vi "Edit_BSA_IP.vi"(3 "Show Panel":bool) -> (1 "Run LDA Diagnostic Out":bool)   [LabVIEW 2017]
uses:
  Controls/Beam_Power.ctl
  BSA_Type.ctl
  File/Setup_Filetype.ctl
  Globals/LDA_meas_global_2.vi
  Globals/LDA_meas_global_1.vi
  Globals/Constants_global.vi
  Globals/Meas_global.vi
panel:
  out "Setup String to read":string
  out "Blue Wavelength":dbl format="%.2f"
  out "Green Wavelength":dbl format="%.2f"
  in  "BSA Type":T1
  in  "45 Degree Mirror":bool
  in  "Beam Alignment":u16(ring) items=["No Info", "Tunnel", "Model"]
  in  "Warn if Power below (mW)":T2
  out "Probe Options":string[](array[string])
  out "Green Fibre Separation":dbl[](array[numeric])
  out "Blue Fibre Separation":dbl[](array[numeric])
  in  "Cluster":cluster{"Focal Lengths":string[]}
  out "Focal Lengths Cluster":cluster{"Focal Lengths":string[]}[](array[cluster])
  out "Channel Values":string[][](array[string])
  out "Channel Names":string[](array[string])
  out "LDA_Probe_Information File":path
  in  "Focal Length 1":u16(ring) items=["160", "300"]
  in  "Focal Length 0":u16(ring) items=["160", "300"]
  in  "Non-coincident":bool=TRUE
  in  "Run LDA Diagnostic":bool
  in  "Bandwidth 0":u16(ring)=11 items=["171.970", "85.985", "42.992", "21.496", "10.748", "5.374", "2.687", "1.344", "0.672", "0.336", "0.168", "0.084"]
  in  "Centre frequency 1":u16(ring)=20 items=["9.563", "8.925", "8.288", "7.650", "7.013", "6.375", "5.738", "5.100", "4.463", "3.825", "3.188", "2.550", "1.913", "1.275", "0.638", "0.000", "-0.638", "-1.275", "-1.913", "-2.550", "-3.188", "-3.825", "-4.463", "-5.100", "-5.738", "-6.375", "-7.013", "-7.650", "-8.288", "-8.925", "-9.563", "-10.200", "-10.838"]
  out "Record Length":dbl[](array[numeric])
  out "Final read?":bool
  in  "OK":bool
  out "C Array":dbl[](array[numeric])
  out "Bandwidth Array Hz":dbl[](array[numeric])
  in  "BSA IP Number":string
  in  "Bandwidth 1":u16(ring)=11 items=["163.205", "81.602", "40.801", "20.401", "10.200", "5.100", "2.550", "1.275", "0.638", "0.319", "0.159", "0.080"]
  in  "Centre frequency 0":u16(ring)=20 items=["10.076", "9.405", "8.733", "8.061", "7.389", "6.718", "6.046", "5.374", "4.702", "4.031", "3.359", "2.687", "2.015", "1.344", "0.672", "0.000", "-0.672", "-1.344", "-2.015", "-2.687", "-3.359", "-4.031", "-4.702", "-5.374", "-6.046", "-6.718", "-7.389", "-8.061", "-8.733", "-9.405", "-10.076", "-10.748", "-11.420"]
  in  "Setup Array":T3(array[cluster]) {"Beams Colour" items=["Green Beams", "Blue Beams"]; "Fibre Colour" items=["Green Fibres", "Blue Fibres"]; "Probe Type" items=["27mm SN141", "27mm SN142", "27mm SN157"]; "Bandwidth Hz" format="%.3g"; "Min Record length" items=["16", "32", "64", "128", "256"]; "Optics Conversion Factor" format="%.3g"; "High voltage" min=0 max=2040 step=8; "Signal gain (dB)" min=0 max=30 step=1; "Max Record length" items=["16", "32", "64", "128", "256"]; "Min Velocity" format="%.2g"; "Max Velocity" format="%.2g"; "Wavelength (nm)" format="%.1f"}
  # "Change wavelength values\nin the LDA _Probe_Info.xls file \nthat lives in the All Users folder \nin the Rig Setup."
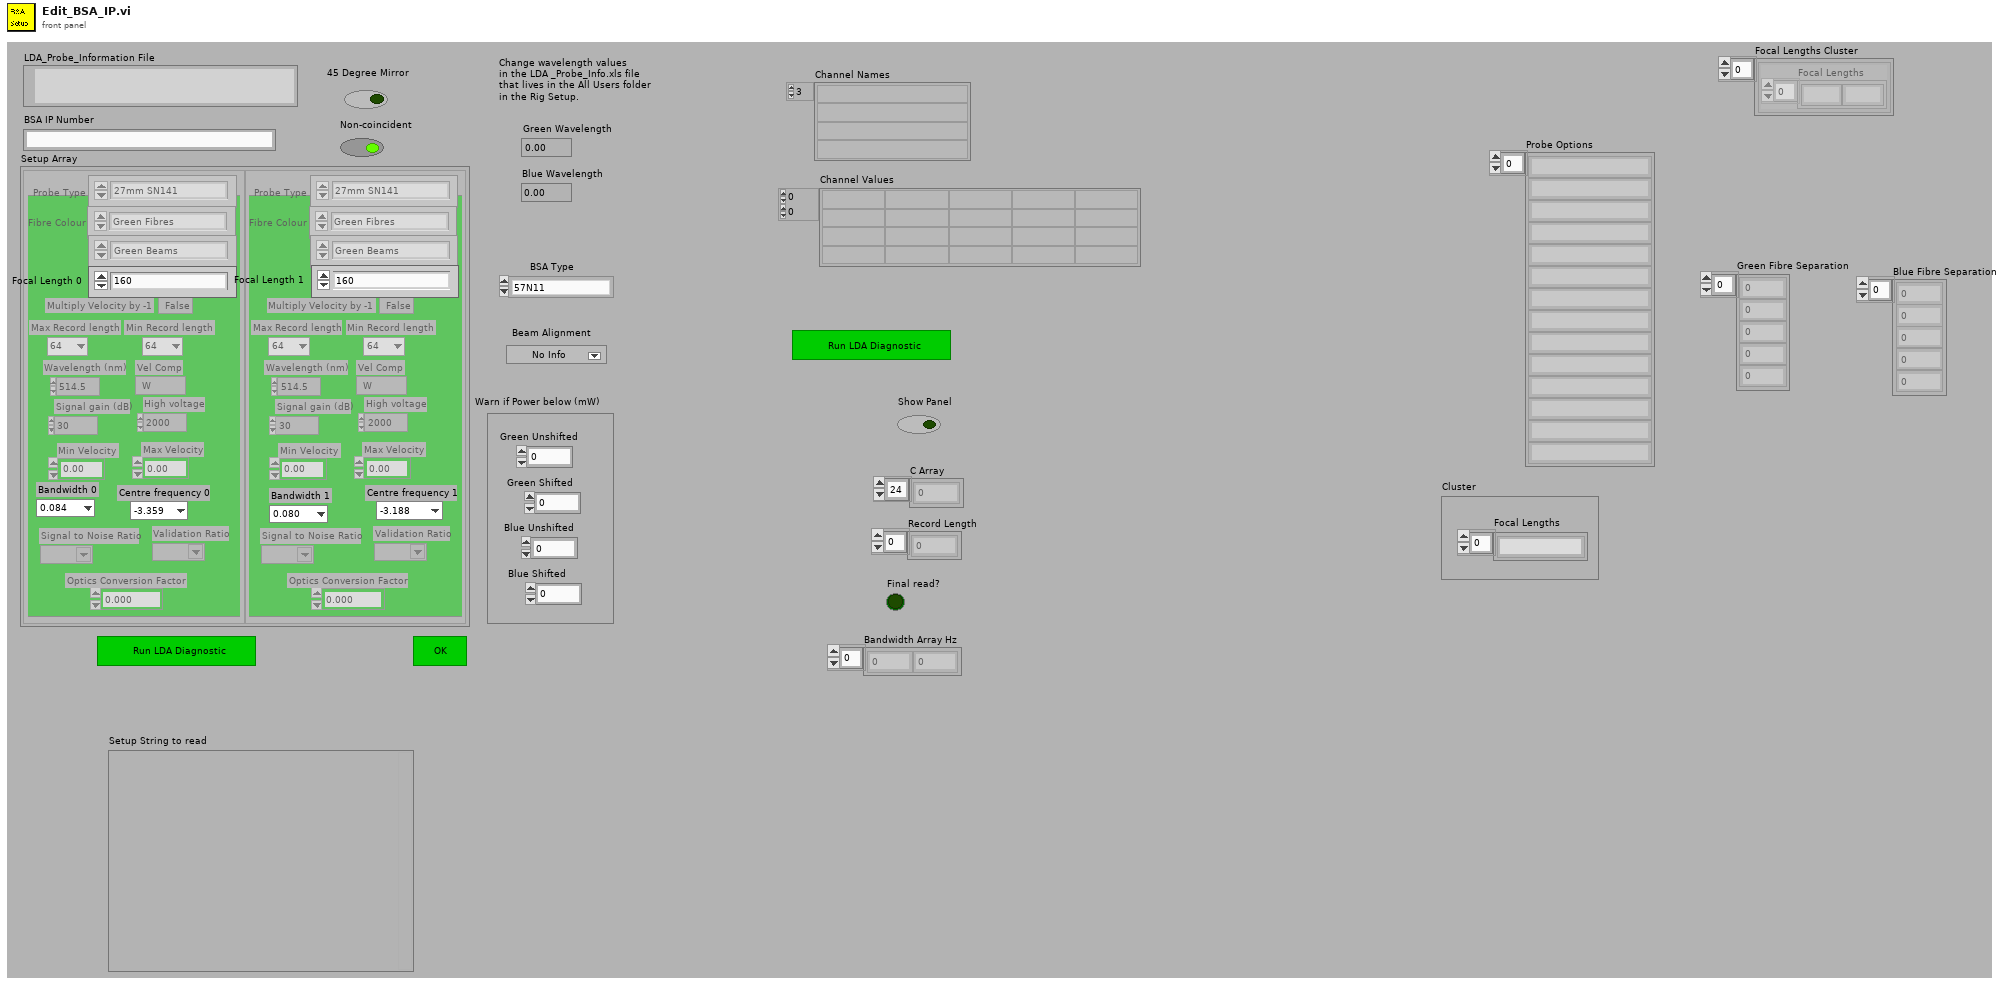
[diagram p1: front panel]
types:
  T1 = typedef "BSA_Type.ctl" = enum16{"57N11", "BSA F60"}
  T2 = typedef "Beam_Power.ctl" = cluster{"Green Unshifted":i32, "Green Shifted":i32, "Blue Unshifted":i32, "Blue Shifted":i32}
  T3 = cluster{"Wavelength (nm)":dbl, "Vel Comp":string, "Max Velocity":dbl, "Min Velocity":dbl, "COLOUR":u32, "Max Record length":u16, "Signal gain (dB)":i16, "High voltage":i16, "Optics Conversion Factor":dbl, "Min Record length":u16, "Bandwidth Hz":dbl, "Multiply Velocity by -1":bool, "Signal to Noise Ratio":string, "Validation Ratio":string, "Probe Type":u16, "Fibre Colour":u16, "Beams Colour":u16}[]
  T4 = typedef "LDA_Setup.ctl" = cluster{"dimensions":enum16{"1D", "2D"}, "Sampling Rate Hz":dbl}
  T5 = typedef "Setup_Filetype.ctl" = enum16{"Measurement Setups", "Calibration Setups", "General", "Results File Plotter Setups", "Speed Calib Tweaks"}
  T6 = cluster{"Wavelength (nm)":dbl, "Vel Comp":string, "Max Velocity":dbl, "Min Velocity":dbl, "COLOUR":u32, "Max Record length":u16, "Signal gain (dB)":i16, "High voltage":i16, "Optics Conversion Factor":dbl, "Min Record length":u16, "Bandwidth Hz":dbl, "Multiply Velocity by -1":bool, "Signal to Noise Ratio":string, "Validation Ratio":string, "Probe Type":u16, "Fibre Colour":u16, "Beams Colour":u16}
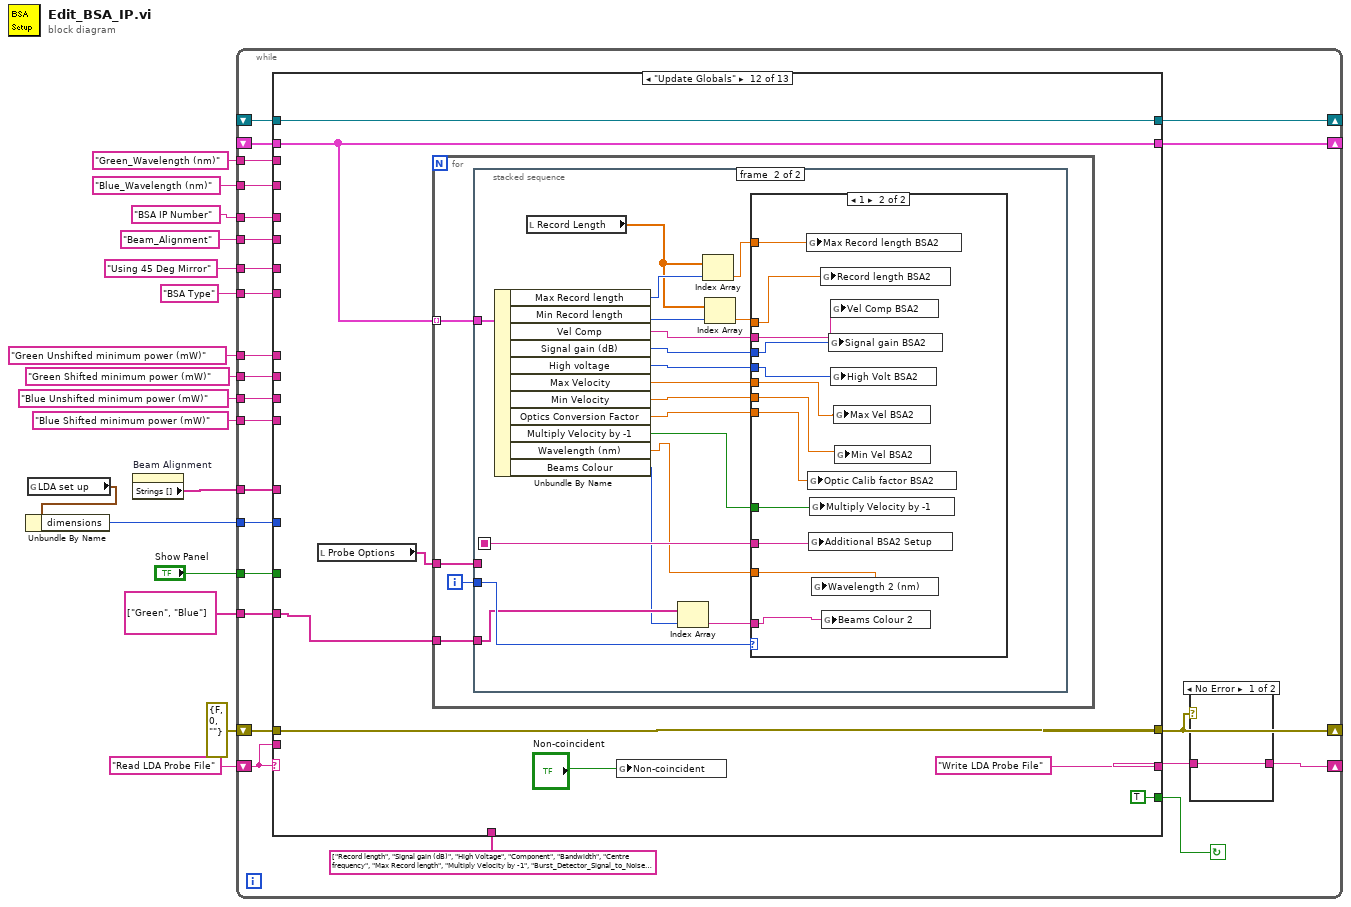
[diagram p0: block diagram]
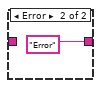
[diagram p2: hidden frame]
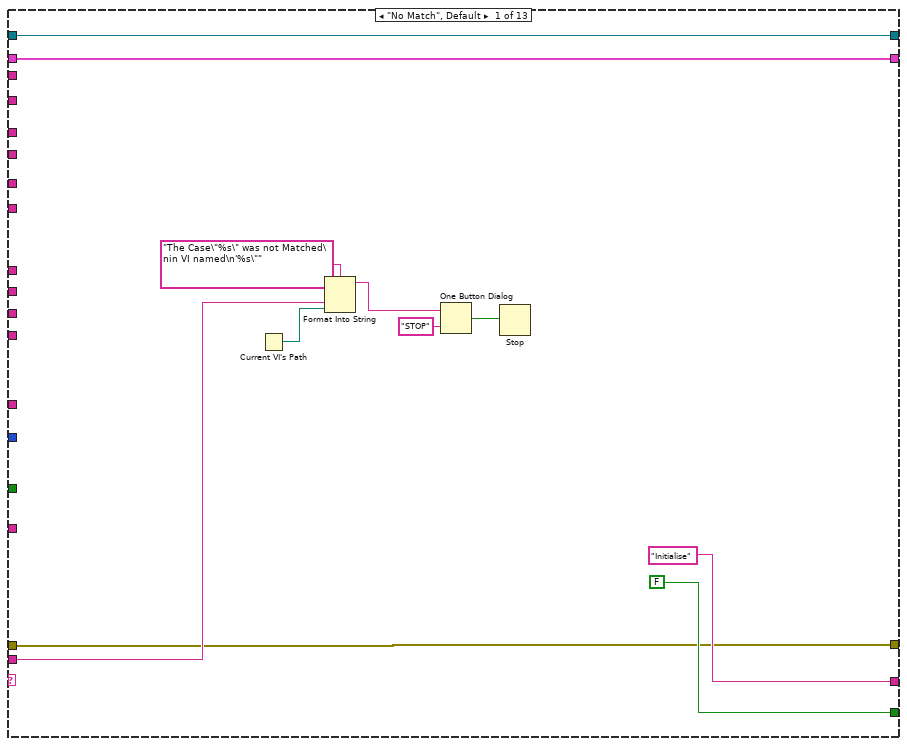
[diagram p3: hidden frame]
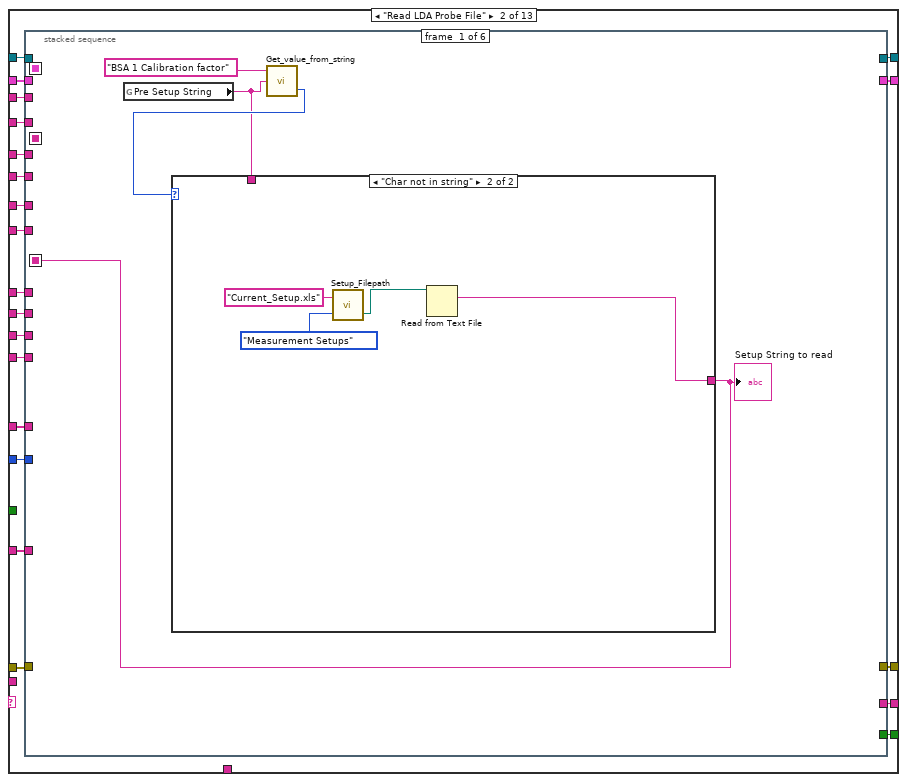
[diagram p4: hidden frame]
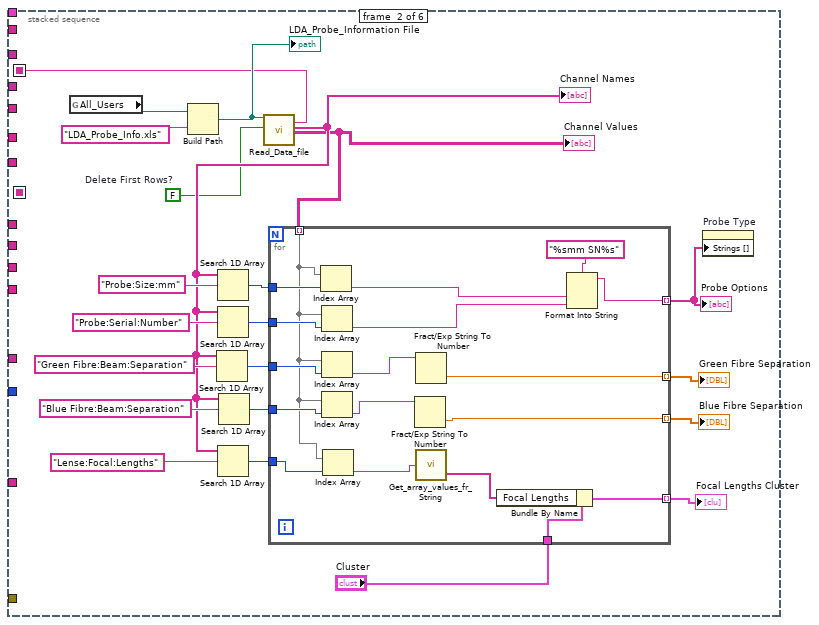
[diagram p6: hidden frame]
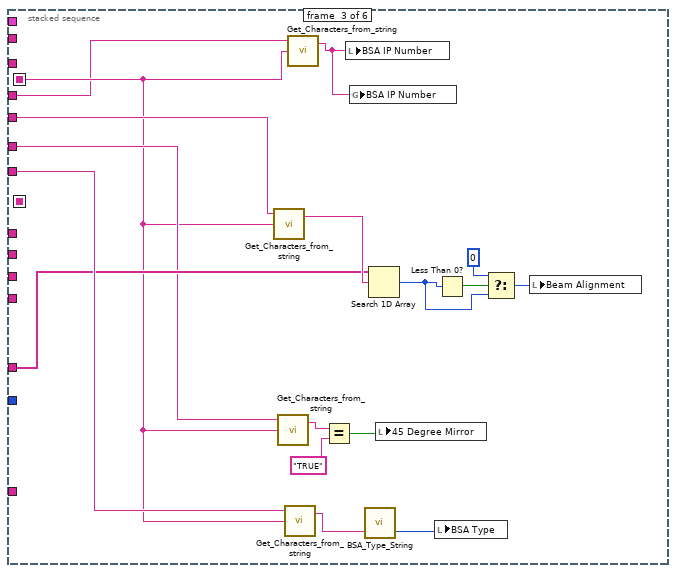
[diagram p7: hidden frame]
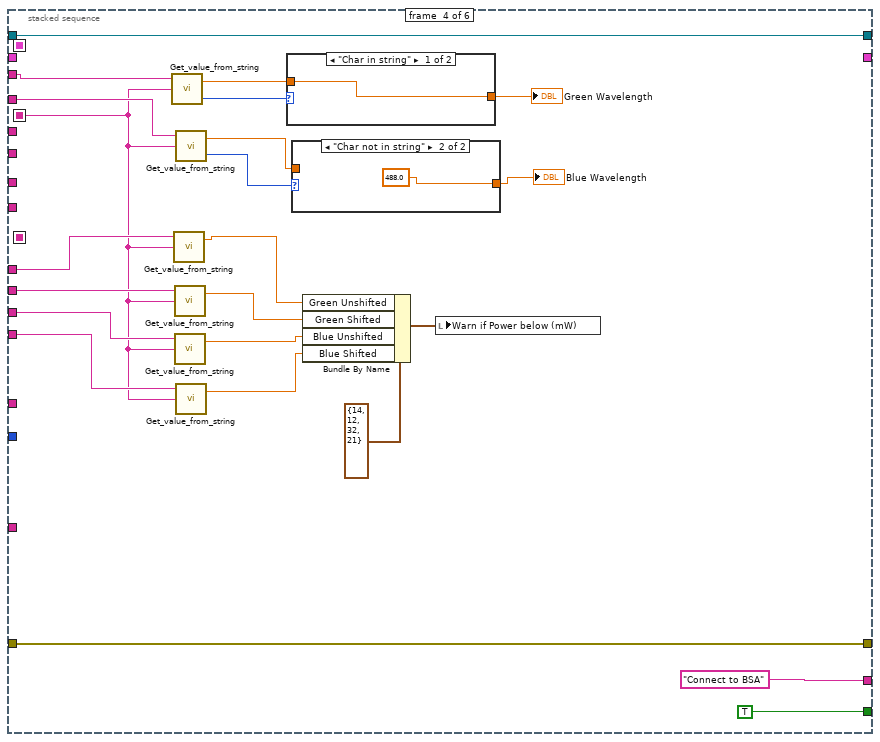
[diagram p8: hidden frame]
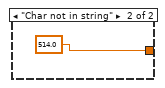
[diagram p10: hidden frame]
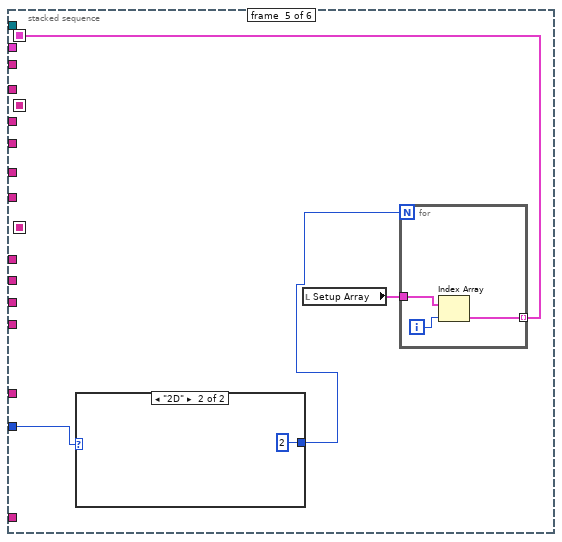
[diagram p11: hidden frame]
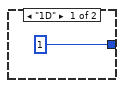
[diagram p12: hidden frame]
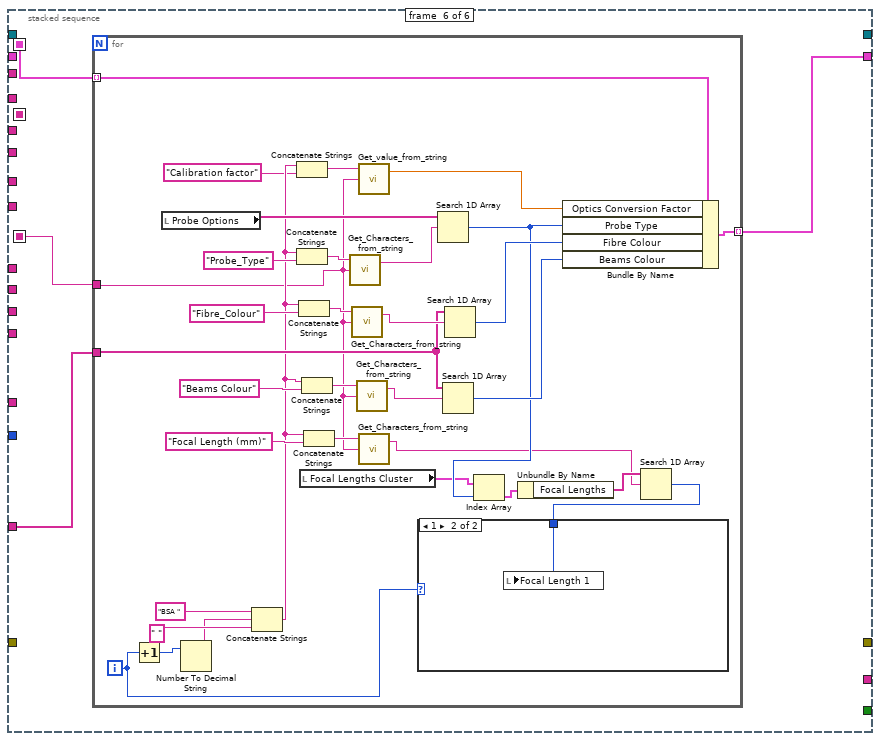
[diagram p13: hidden frame]
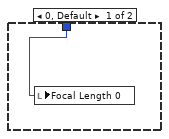
[diagram p14: hidden frame]
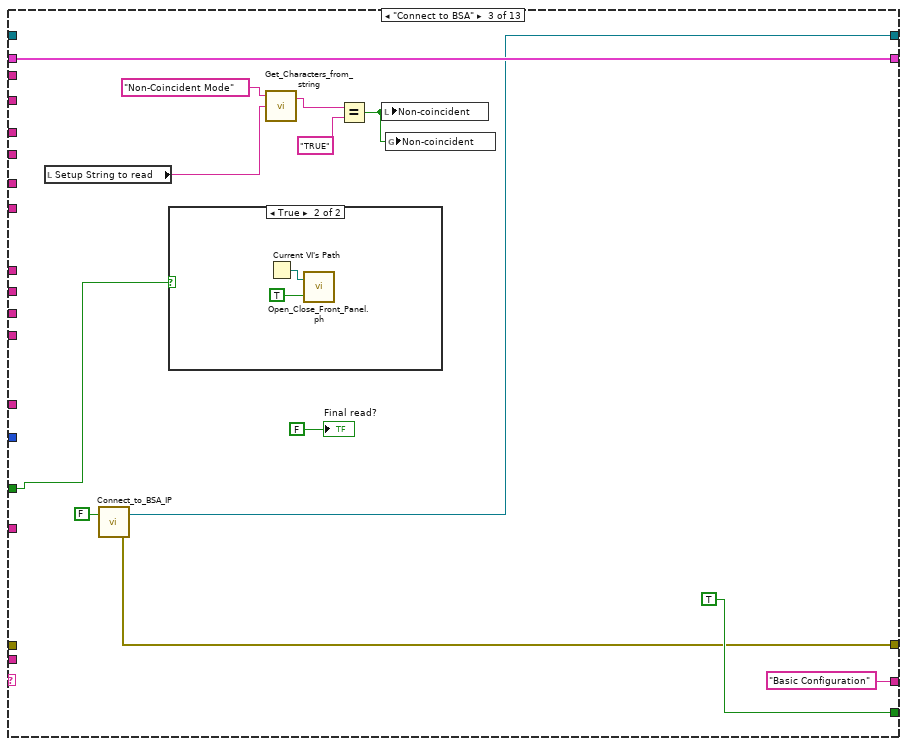
[diagram p15: hidden frame]
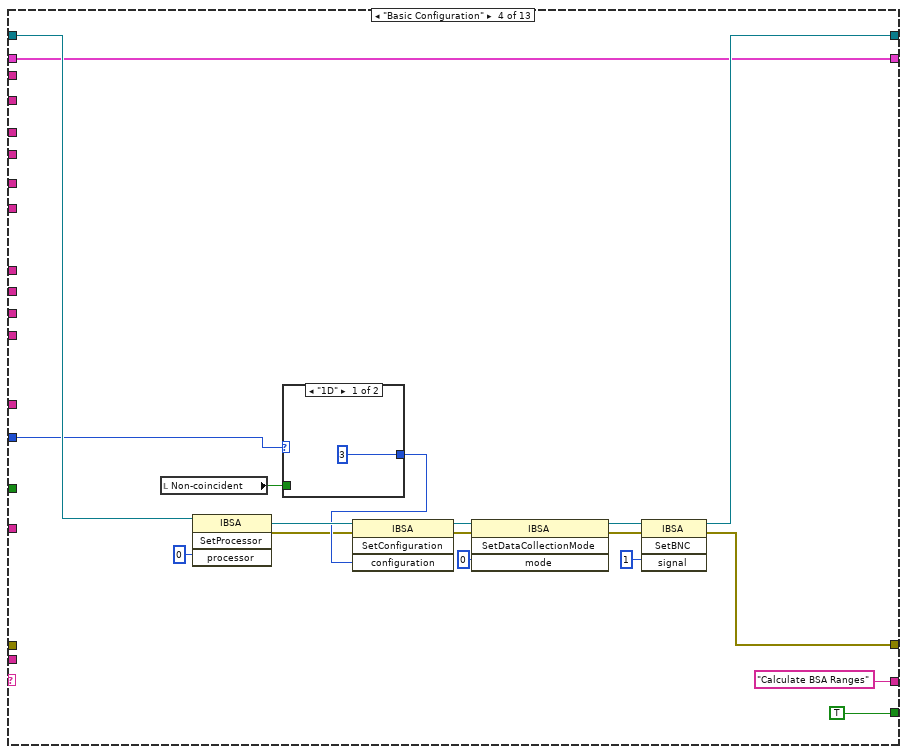
[diagram p17: hidden frame]
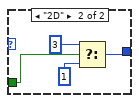
[diagram p18: hidden frame]
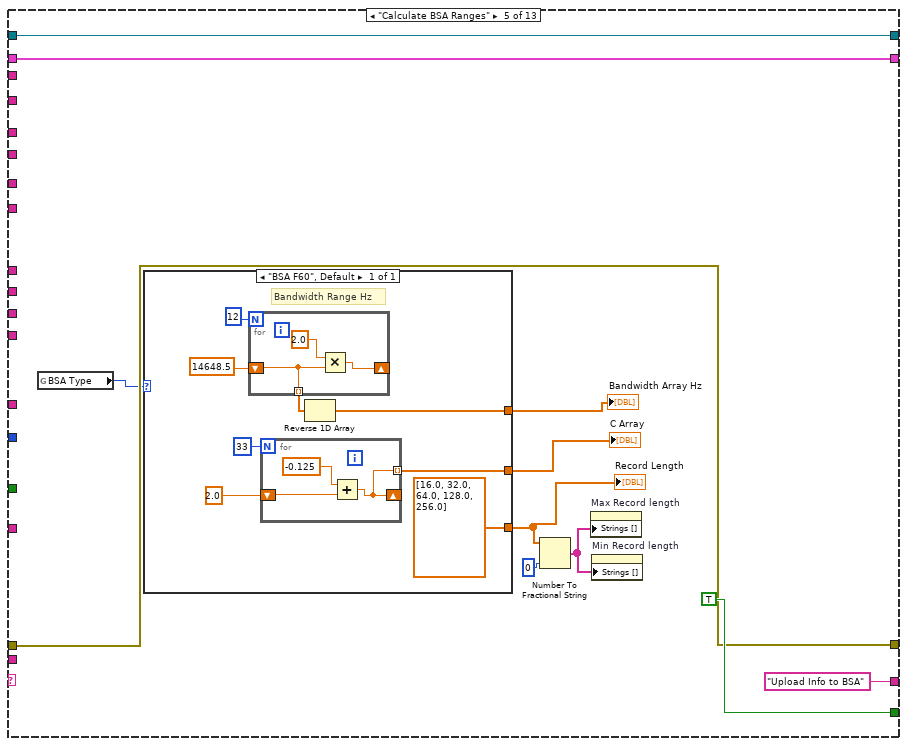
[diagram p19: hidden frame]
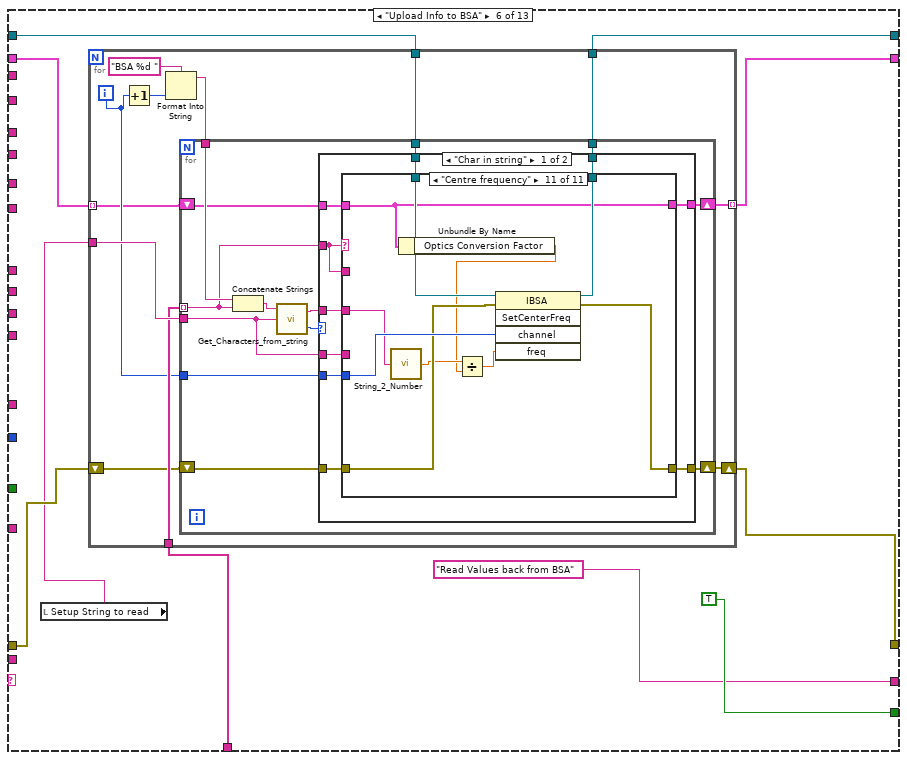
[diagram p20: hidden frame]
diagram:
  n1 = global read "Meas_global.vi" "LDA set up"() -> (w5:T4)
  n2 = Unbundle By Name(w5) -> ("dimensions"=w4:enum16{"1D", "2D"})
  n3 = property on="Beam Alignment" class="Ring (strict)"() -> ("Strings []"=w7:string[])  [unwired: 2 in, 2 out]
  n4 = while {
    shift-left: "Read LDA Probe File" -> [w41]
    shift-right: [w40] -> _
    shift-right: [w38] -> _
    shift-left: _ -> [w36]
    shift-right: [w31] -> _
    shift-left: errorcluster {"status"=FALSE, "code"=0, "source"=""} ("error out") -> [w37]
    shift-right: [w35] -> _
    shift-left: _ -> [w34]
    tunnel: "Show Panel" -> [w32]
    tunnel: "Green Unshifted minimum power (mW)" -> [w30]
    tunnel: "Green Shifted minimum power (mW)" -> [w29]
    tunnel: "Blue Unshifted minimum power (mW)" -> [w28]
    tunnel: "Blue Shifted minimum power (mW)" -> [w27]
    tunnel: "Using 45 Deg Mirror" -> [w26]
    tunnel: "BSA Type" -> [w25]
    tunnel: "Beam_Alignment" -> [w24]
    tunnel: "BSA IP Number" -> [w23]
    tunnel: w7 -> [w22]
    tunnel: string[] ["Green", "Blue"] -> [w21]
    tunnel: w4 -> [w20]
    tunnel: "Green_Wavelength (nm)" -> [w19]
    tunnel: "Blue_Wavelength (nm)" -> [w18]
    stop <- w42 continue-if-true
    n5 = case shown="\"Update Globals\"" w41 {
      tunnel: [FALSE w75 TRUE TRUE TRUE TRUE TRUE TRUE TRUE ("Show Panel") TRUE TRUE TRUE ("Show Panel") w931] -> w42
      tunnel: ["Initialise" w76 "Basic Configuration" "Calculate BSA Ranges" "Upload Info to BSA" "Read Values back from BSA" w428 w565 w690 "Read Values back from BSA" "Update Globals" ("t") "Write LDA Probe File" w928] -> w39
      tunnel: w41 -> [w50 _ _ _ _ _ _ _ _ _ _ _ _]
      tunnel: [w46 w73 w226 w237 w263 w286 w435 w570 w692 w711 errorcluster {"status"=FALSE, "code"=0, "source"=""} ("error out") w834 w929] -> w31
      tunnel: [w47 w71 w227 w239 w265 w288 w437 w575 w696 w713 w826 w836 w924] -> w38
      tunnel: w37 -> [w46 w74 _ _ w263 w287 w436 w570 w692 w712 w825 w834 w930]
      tunnel: w36 -> [w47 w72 _ w245 w265 w289 w438 w575 w696 w714 w826 w836 w925]
      tunnel: [w45 w70 w228 w233 w264 w284 w432 w571 w689 w709 w824 w835 w926] -> w35
      tunnel: w34 -> [w45 w69 w228 w233 w264 w285 w434 _ w689 w710 w824 w835 w927]
      tunnel: string[] ["Record length", "Signal gain (dB)", "High Voltage", "Component", "Bandwidth", "Centre frequency", "Max Record length", "Multiply Velocity by -1", "Burst_Detector_Signal_to_Noise_Ratio", "Level_Validation_Ratio"] -> [_ _ _ _ _ w283 w433 _ _ w708 _ _ _]
      tunnel: w32 -> [_ _ w224 _ _ _ _ w562 _ _ _ _ w914]
      tunnel: w30 -> [_ w68 _ _ _ _ _ _ _ _ _ _ w923]
      tunnel: w29 -> [_ w67 _ _ _ _ _ _ _ _ _ _ w922]
      tunnel: w28 -> [_ w66 _ _ _ _ _ _ _ _ _ _ w921]
      tunnel: w27 -> [_ w65 _ _ _ _ _ _ _ _ _ _ w920]
      tunnel: w26 -> [_ w61 _ _ _ _ _ _ _ _ _ _ w919]
      tunnel: w25 -> [_ w64 _ _ _ _ _ _ _ _ _ _ w918]
      tunnel: w24 -> [_ w63 _ _ _ _ _ _ _ _ _ _ w917]
      tunnel: w23 -> [_ w60 _ _ _ _ _ _ _ _ _ _ w916]
      tunnel: w22 -> [_ w62 _ _ _ _ _ _ _ _ _ _ w915]
      tunnel: w21 -> [_ w59 _ _ _ _ _ _ _ _ _ w829 _]
      tunnel: w20 -> [_ w58 _ w234 _ _ _ _ _ _ _ _ _]
      tunnel: w19 -> [_ w56 _ _ _ _ _ _ _ _ _ _ w913]
      tunnel: w18 -> [_ w57 _ _ _ _ _ _ _ _ _ _ w912]
      frame "No Match", Default {
        n6 = Current VI's Path() -> (path=w49:path)
        n7 = Format Into String(format string="The Case\"%s\" was not Matched\nin VI named\n'%s\"" ("Format String"), w50, w49) -> (resulting string=w53:string)  [unwired: 2 in, 1 out]
        n8 = One Button Dialog(message=w53, button name ("OK")="STOP") -> (true=w51:bool)
        n9 = Stop(stop? (T)=w51) -> ()
      }
      frame "Read LDA Probe File" {
        n10 = stacked-sequence {
          seq-local: [_ w104 _ _ _ _] -> [_ _ w128 w149 _ _]
          seq-local: [_ _ _ _ w170 _] -> [_ _ _ _ _ w180]
          seq-local: [w78 _ _ _ _ _] -> [_ _ _ _ _ w179]
          tunnel: [_ _ _ "Connect to BSA" _ _] -> w76
          tunnel: [_ _ _ TRUE ("Show Panel") _ _] -> w75
          tunnel: w74 -> [_ _ _ w163 _ _]
          tunnel: [_ _ _ w163 _ _] -> w73
          tunnel: w72 -> [_ _ _ w162 _ _]
          tunnel: [_ _ _ w162 _ _] -> w71
          tunnel: [_ _ _ _ _ w181] -> w70
          tunnel: w69 -> [_ _ _ _ _ _]
          tunnel: w68 -> [_ _ _ w155 _ _]
          tunnel: w67 -> [_ _ _ w154 _ _]
          tunnel: w66 -> [_ _ _ w153 _ _]
          tunnel: w65 -> [_ _ _ w152 _ _]
          tunnel: w64 -> [_ _ w140 _ _ _]
          tunnel: w63 -> [_ _ w135 _ _ _]
          tunnel: w62 -> [_ _ w134 _ _ _]
          tunnel: w61 -> [_ _ w130 _ _ _]
          tunnel: w60 -> [_ _ w127 _ _ _]
          tunnel: w59 -> [_ _ _ _ _ w182]
          tunnel: w58 -> [_ _ _ _ w172 _]
          tunnel: w57 -> [_ _ _ w151 _ _]
          tunnel: w56 -> [_ _ _ w150 _ _]
          frame #0 {
            n11 = global read "Meas_global.vi" "Pre Setup String"() -> (w77:string)
            n12 = call "Get_value_from_string.vi"("Input string"=w77, "Variable name"="BSA 1 Calibration factor") -> ("Status"=w79:enum16{"Char in string", "Char not in string"})  [unwired: 1 in, 1 out]
            n13 = case shown="\"Char not in string\"" w79 {
              tunnel: [w81 w82] -> w78
              tunnel: w77 -> [w81 _]
              frame "Char in string" {
              }
              frame "Char not in string" {
                n14 = call "Setup_Filepath.vi"("Setup File Type"=Setup_Filetype."Measurement Setups", "Filename in"="Current_Setup.xls") -> ("Filename Out"=w83:path)  [unwired: 1 out]
                n15 = Read from Text File(file (use dialog)=w83) -> (text=w82:string)  [unwired: 3 in, 3 out]
              }
            }
            "Setup String to read" <- w78
          }
          frame #1 {
            w86 = FALSE  # Delete First Rows?
            n16 = global read "Constants_global.vi" "All_Users"() -> (w107:path)
            n17 = Build Path(base path=w107, name or relative path="LDA_Probe_Info.xls") -> (appended path=w105:path)
            "LDA_Probe_Information File" <- w105
            n18 = call "Read_Data_file.vi"("Results file"=w105, "Delete First Rows?"=w86) -> ("String Before"=w104:string, "Ch names Out"=w89:string[], "Channel Values Out"=w88:string[][])  [unwired: 7 in, 8 out]
            "Channel Names" <- w89
            "Channel Values" <- w88
            n19 = Search 1D Array(1D array=w89, element="Green Fibre:Beam:Separation") -> (index of element=w97:i32)  [unwired: 1 in]
            n20 = Search 1D Array(1D array=w89, element="Probe:Size:mm") -> (index of element=w92:i32)  [unwired: 1 in]
            n21 = Search 1D Array(1D array=w89, element="Probe:Serial:Number") -> (index of element=w93:i32)  [unwired: 1 in]
            n22 = Search 1D Array(1D array=w89, element="Lense:Focal:Lengths") -> (index of element=w101:i32)  [unwired: 1 in]
            n23 = Search 1D Array(1D array=w89, element="Blue Fibre:Beam:Separation") -> (index of element=w96:i32)  [unwired: 1 in]
            n24 = for {
              tunnel: w92 -> [w125]
              tunnel: w88 -> [w113] mode=indexing
              tunnel: w93 -> [w124]
              tunnel: [w120] -> w87 mode=indexing
              tunnel: w96 -> [w119]
              tunnel: w97 -> [w118]
              tunnel: [w115] -> w98 mode=indexing
              tunnel: [w114] -> w99 mode=indexing
              tunnel: w101 -> [w112]
              tunnel: "Cluster" -> [w110]
              tunnel: [w108] -> w103 mode=indexing
              n25 = Index Array(array=w113, index=w125) -> (element=w122:string)
              n26 = Index Array(array=w113, index=w124) -> (element=w121:string)
              n27 = Index Array(array=w113, index=w118) -> (element=w117:string)
              n28 = Index Array(array=w113, index=w119) -> (element=w116:string)
              n29 = Index Array(array=w113, index=w112) -> (element=w111:string)
              n30 = Fract/Exp String To Number(string=w116) -> (number=w114:dbl)  [unwired: 3 in, 1 out]
              n31 = Fract/Exp String To Number(string=w117) -> (number=w115:dbl)  [unwired: 3 in, 1 out]
              n32 = call "Get_array_values_fr_String.vi"("String Value"=w111) -> ("String array"=w109:string[])  [unwired: 1 out]
              n33 = Bundle By Name(cluster=w110, "Focal Lengths"=w109) -> (w108:cluster{"Focal Lengths":string[]})
              n34 = Format Into String(format string="%smm SN%s", w122, w121) -> (resulting string=w120:string)  [unwired: 2 in, 1 out]
            }
            "Probe Options" <- w87
            "Green Fibre Separation" <- w98
            "Blue Fibre Separation" <- w99
            "Focal Lengths Cluster" <- w103
            n35 = property on="Probe Type" class="Ring (strict)"("Strings []"=w87) -> ()  [unwired: 2 in, 2 out]
          }
          frame #2 {
            n36 = call "Get_Characters_from_string.vi"("Input string"=w128, "Variable name"=w135) -> ("Value"=w136:string)  [unwired: 1 in, 1 out]
            n37 = call "Get_Characters_from_string.vi"("Input string"=w128, "Variable name"=w130) -> ("Value"=w131:string)  [unwired: 1 in, 1 out]
            n38 = call "Get_Characters_from_string.vi"("Input string"=w128, "Variable name"=w140) -> ("Value"=w142:string)  [unwired: 1 in, 1 out]
            n39 = call "Get_Characters_from_string.vi"("Input string"=w128, "Variable name"=w127) -> ("Value"=w126:string)  [unwired: 1 in, 1 out]
            n40 = Equal?(x=w131, y="TRUE") -> (x = y?=w129:bool)
            n41 = local write "BSA IP Number"(w126) -> ()
            n42 = global write "LDA_meas_global_1.vi" "BSA IP Number"(w126) -> ()
            n43 = call "BSA_Type_String.vi"("BSA String in"=w142) -> ("BSA Type Out"=w141:T1)  [unwired: 1 in, 1 out]
            n44 = Search 1D Array(1D array=w134, element=w136) -> (index of element=w139:i32)  [unwired: 1 out]
            n45 = local write "45 Degree Mirror"(w129) -> ()
            n46 = local write "BSA Type"(w141) -> ()
            n47 = Less Than 0?(x=w139) -> (x < 0?=w137:bool)
            n48 = Select(t=0, s=w137, f=w139) -> (s? t:f=w133:i32)
            n49 = local write "Beam Alignment"(w133) -> ()
          }
          frame #3 {
            n50 = call "Get_value_from_string.vi"("Input string"=w149, "Variable name"=w150) -> ("Status"=w148:enum16{"Char in string", "Char not in string"}, "Value"=w146:dbl)  [unwired: 1 in]
            n51 = call "Get_value_from_string.vi"("Input string"=w149, "Variable name"=w155) -> ("Value"=w161:dbl)  [unwired: 1 in, 1 out]
            n52 = call "Get_value_from_string.vi"("Input string"=w149, "Variable name"=w154) -> ("Value"=w158:dbl)  [unwired: 1 in, 1 out]
            n53 = call "Get_value_from_string.vi"("Input string"=w149, "Variable name"=w153) -> ("Value"=w159:dbl)  [unwired: 1 in, 1 out]
            n54 = call "Get_value_from_string.vi"("Input string"=w149, "Variable name"=w151) -> ("Status"=w144:enum16{"Char in string", "Char not in string"}, "Value"=w145:dbl)  [unwired: 1 in]
            n55 = call "Get_value_from_string.vi"("Input string"=w149, "Variable name"=w152) -> ("Value"=w160:dbl)  [unwired: 1 in, 1 out]
            n56 = case shown="\"Char in string\"" w148 {
              tunnel: [w168 514.0 ("Wavelength (nm)")] -> w147
              tunnel: w146 -> [w168 _]
              frame "Char in string" {
              }
              frame "Char not in string" {
              }
            }
            "Green Wavelength" <- w147
            n57 = case shown="\"Char not in string\"" w144 {
              tunnel: [w166 488.0 ("Wavelength (nm)")] -> w143
              tunnel: w145 -> [w166 _]
              frame "Char in string" {
              }
              frame "Char not in string" {
              }
            }
            "Blue Wavelength" <- w143
            n58 = Bundle By Name(cluster=T2 {"Green Unshifted"=14, "Green Shifted"=12, "Blue Unshifted"=32, "Blue Shifted"=21} ("Warn if Power below (mW)"), "Green Unshifted"=w161, "Green Shifted"=w158, "Blue Unshifted"=w159, "Blue Shifted"=w160) -> (w157:T2)
            n59 = local write "Warn if Power below (mW)"(w157) -> ()
          }
          frame #4 {
            n60 = case shown="\"2D\"" w172 {
              tunnel: [1 2] -> w171
              frame "1D" {
              }
              frame "2D" {
              }
            }
            n61 = local read "Setup Array"() -> (w173:T3)
            n62 = for {
              N: w171 -> [_]
              tunnel: w173 -> [w177]
              tunnel: [w176] -> w170 mode=indexing
              i -> [w178]
              n63 = Index Array(array=w177, index=w178) -> (element=w176:T6)
            }
          }
          frame #5 {
            n64 = for {
              tunnel: w180 -> [w211] mode=indexing
              tunnel: w179 -> [w185]
              tunnel: w182 -> [w200]
              tunnel: [w188] -> w181 mode=indexing
              i -> [w197]
              n65 = Increment(x=w197) -> (x+1=w214:i32)
              n66 = local read "Probe Options"() -> (w208:string[])
              n67 = Number To Decimal String(number=w214) -> (decimal integer string=w212:string)  [unwired: 1 out]
              n68 = Concatenate Strings("BSA ", w212, " ") -> (w187:string)
              n69 = Concatenate Strings(w187, "Calibration factor") -> (w184:string)
              n70 = Concatenate Strings(w187, "Probe_Type" ("Pre Setup String")) -> (w209:string)
              n71 = Concatenate Strings(w187, "Fibre_Colour" ("string")) -> (w206:string)
              n72 = local read "Focal Lengths Cluster"() -> (w194:cluster{"Focal Lengths":string[]}[])
              n73 = Concatenate Strings(w187, "Beams Colour") -> (w201:string)
              n74 = Concatenate Strings(w187, "Focal Length (mm)") -> (w193:string)
              n75 = call "Get_Characters_from_string.vi"("Input string"=w185, "Variable name"=w209) -> ("Value"=w207:string)  [unwired: 1 in, 1 out]
              n76 = call "Get_Characters_from_string.vi"("Input string"=w185, "Variable name"=w206) -> ("Value"=w204:string)  [unwired: 1 in, 1 out]
              n77 = call "Get_Characters_from_string.vi"("Input string"=w185, "Variable name"=w201) -> ("Value"=w199:string)  [unwired: 1 in, 1 out]
              n78 = call "Get_value_from_string.vi"("Input string"=w185, "Variable name"=w184) -> ("Value"=w183:dbl)  [unwired: 1 in, 1 out]
              n79 = call "Get_Characters_from_string.vi"("Input string"=w185, "Variable name"=w193) -> ("Value"=w190:string)  [unwired: 1 in, 1 out]
              n80 = Search 1D Array(1D array=w208, element=w207) -> (index of element=w195:i32)  [unwired: 1 in]
              n81 = Search 1D Array(1D array=w200, element=w199) -> (index of element=w198:i32)  [unwired: 1 in]
              n82 = Search 1D Array(1D array=w200, element=w204) -> (index of element=w203:i32)  [unwired: 1 in]
              n83 = Index Array(array=w194, index=w195) -> (element=w196:cluster{"Focal Lengths":string[]})
              n84 = Unbundle By Name(w196) -> ("Focal Lengths"=w191:string[])
              n85 = Bundle By Name(cluster=w211, "Optics Conversion Factor"=w183, "Probe Type"=w195, "Fibre Colour"=w203, "Beams Colour"=w198) -> (w188:T6)
              n86 = Search 1D Array(1D array=w191, element=w190) -> (index of element=w189:i32)  [unwired: 1 in]
              n87 = case shown="1" w197 {
                tunnel: w189 -> [w216 w217]
                frame 0, Default {
                  n88 = local write "Focal Length 0"(w216) -> ()
                }
                frame 1 {
                  n89 = local write "Focal Length 1"(w217) -> ()
                }
              }
            }
          }
        }
      }
      frame "Connect to BSA" {
        n90 = local read "Setup String to read"() -> (w218:string)
        n91 = call "Connect_to_BSA_IP.vi"("Force Reconnect"=FALSE) -> ("error out"=w226:errorcluster, "BSA"=w227:refnum<k7>)  [unwired: 1 out]
        n92 = case shown="True" w224 {
          frame False {
          }
          frame True {
            n93 = Current VI's Path() -> (path=w231:path)
            n94 = call "Open_Close_Front_Panel.ph.vi"("Front Panel Window:Open"=TRUE, "VI path"=w231) -> ()  [unwired: 2 out]
          }
        }
        n95 = call "Get_Characters_from_string.vi"("Input string"=w218, "Variable name"="Non-Coincident Mode" ("Pre Setup String")) -> ("Value"=w222:string)  [unwired: 1 in, 1 out]
        n96 = Equal?(x=w222, y="TRUE") -> (x = y?=w220:bool)
        n97 = local write "Non-coincident"(w220) -> ()
        n98 = global write "LDA_meas_global_1.vi" "Non-coincident"(w220) -> ()
        "Final read?" <- FALSE ("Boolean")
      }
      frame "Basic Configuration" {
        n99 = local read "Non-coincident"() -> (w241:bool)
        n100 = invoke class="IBSA" method="SetProcessor"(reference=w245, "processor"=0) -> (reference out=w248:refnum<k7>, error out=w246:errorcluster)  [unwired: 2 in, 2 out]
        n101 = case shown="\"1D\"" w234 {
          tunnel: [3 ("config") w255] -> w247
          tunnel: w241 -> [_ w254]
          frame "1D" {
          }
          frame "2D" {
            n102 = Select(t=3, s=w254, f=1 ("config")) -> (s? t:f=w255:i32)
          }
        }
        n103 = invoke class="IBSA" method="SetConfiguration"(reference=w248, error in=w246, "configuration"=w247) -> (reference out=w244:refnum<k7>, error out=w243:errorcluster)  [unwired: 1 in, 2 out]
        n104 = invoke class="IBSA" method="SetDataCollectionMode"(reference=w244, error in=w243, "mode"=0) -> (reference out=w240:refnum<k7>, error out=w238:errorcluster)  [unwired: 1 in, 2 out]
        n105 = invoke class="IBSA" method="SetBNC"(reference=w240, error in=w238, "signal"=1) -> (reference out=w239:refnum<k7>, error out=w237:errorcluster)  [unwired: 1 in, 2 out]
      }
      frame "Calculate BSA Ranges" {
        n106 = global read "LDA_meas_global_1.vi" "BSA Type"() -> (w257:T1)
        n107 = case shown="\"BSA F60\", Default" w257 {
          tunnel: [w269] -> w261
          tunnel: [w268] -> w260
          tunnel: [dbl[] [16.0, 32.0, 64.0, 128.0, 256.0] ("Max Record Length")] -> w258
          frame "BSA F60", Default {
            # "Bandwidth Range Hz"
            n108 = for {
              N: 12 -> [_]
              shift-right: [w280] -> _
              shift-left: 14648.5 -> [w278]
              tunnel: [w278] -> w272 mode=indexing
              n109 = Multiply(x=2.0, y=w278) -> (x*y=w280:dbl)
            }
            n110 = for {
              N: 33 -> [_]
              shift-right: [w275] -> _
              shift-left: 2.0 -> [w277]
              tunnel: [w275] -> w269 mode=indexing
              n111 = Add(x=-0.125, y=w277) -> (x+y=w275:dbl)
            }
            n112 = Reverse 1D Array(array=w272) -> (reversed array=w268:dbl[])
          }
        }
        "C Array" <- w261
        "Bandwidth Array Hz" <- w260
        "Record Length" <- w258
        n113 = Number To Fractional String(number=w258, precision (6)=i16 0) -> (F-format string=w256:string[])  [unwired: 2 out]
        n114 = property on="Max Record length" class="Ring (strict)"("Strings []"=w256) -> ()  [unwired: 2 in, 2 out]
        n115 = property on="Min Record length" class="Ring (strict)"("Strings []"=w256) -> ()  [unwired: 2 in, 2 out]
      }
      frame "Upload Info to BSA" {
        n116 = local read "Setup String to read"() -> (w281:string)
        n117 = for {
          tunnel: w281 -> [w302]
          tunnel: w289 -> [w301]
          tunnel: [w300] -> w288
          shift-right: [w297] -> w286
          shift-left: w287 -> [w298]
          tunnel: w283 -> [w299]
          tunnel: w285 -> [w292] mode=indexing
          tunnel: [w291] -> w284 mode=indexing
          i -> [w296]
          n118 = Increment(x=w296) -> (x+1=w295:i32)
          n119 = Format Into String(format string="BSA %d ", w295) -> (resulting string=w293:string)  [unwired: 2 in, 1 out]
          n120 = for {
            tunnel: w293 -> [w315]
            tunnel: w296 -> [w314]
            tunnel: w302 -> [w307]
            tunnel: w301 -> [w313]
            tunnel: [w312] -> w300
            tunnel: w299 -> [w311] mode=indexing
            shift-right: [w309] -> w297
            shift-left: w298 -> [w310]
            shift-right: [w303] -> w291
            shift-left: w292 -> [w304]
            n121 = Concatenate Strings(w315, w311) -> (w308:string)
            n122 = call "Get_Characters_from_string.vi"("Input string"=w307, "Variable name"=w308) -> ("Status"=w306:enum16{"Char in string", "Char not in string"}, "Value"=w305:string)  [unwired: 1 in]
            n123 = case shown="\"Char in string\"" w306 {
              tunnel: w314 -> [w325 _]
              tunnel: w305 -> [w324 _]
              tunnel: w311 -> [w319 _]
              tunnel: w313 -> [w323 w426]
              tunnel: [w322 w426] -> w312
              tunnel: [w321 w425] -> w309
              tunnel: w310 -> [w320 w425]
              tunnel: w304 -> [w318 w424]
              tunnel: w307 -> [w317 _]
              tunnel: [w316 w424] -> w303
              frame "Char in string" {
                n124 = case shown="\"Centre frequency\"" w319 {
                  tunnel: w325 -> [_ w336 w346 w363 w371 w377 w386 w394 _ w413 w423]
                  tunnel: w324 -> [_ w339 w350 w358 w365 w379 w384 w392 w401 w408 w418]
                  tunnel: w323 -> [w333 w341 w352 w362 w370 w373 w388 w396 w397 w412 w422]
                  tunnel: [w333 w335 w342 w361 w369 w374 w381 w389 w397 w411 w421] -> w322
                  tunnel: [w332 w334 w343 w360 w368 w375 w382 w390 w398 w410 w420] -> w321
                  tunnel: w320 -> [w332 w340 w351 w359 w367 w372 w387 w395 w398 w409 w419]
                  tunnel: w319 -> [w331 _ _ _ _ _ _ _ _ _ _]
                  tunnel: w318 -> [w326 w338 w349 w357 w364 w380 w385 w393 w403 w406 w416]
                  tunnel: w317 -> [_ _ _ _ _ _ _ _ _ _ _]
                  tunnel: [w326 w338 w349 w357 w364 w378 w385 w393 w402 w406 w416] -> w316
                  frame "No Match", Default {
                    n125 = Concatenate Strings(w331, " has not been matched" ("string")) -> (w329:string)
                    n126 = One Button Dialog(message=w329, button name ("OK")="Stop") -> (true=w327:bool)
                    n127 = Stop(stop? (T)=w327) -> ()
                  }
                  frame "Record length" {
                    n128 = Decimal String To Number(string=w339) -> (number=w337:i32)  [unwired: 3 out]
                    n129 = invoke class="IBSA" method="SetRecordLength"(reference=w341, error in=w340, "channel"=w336, "length"=w337) -> (reference out=w335:refnum<k7>, error out=w334:errorcluster)  [unwired: 1 in, 3 out]
                  }
                  frame "Max Record length" {
                    n130 = Decimal String To Number(string=w350) -> (number=w348:i32)  [unwired: 3 out]
                    n131 = invoke class="IBSA" method="SetMaxRecordLength"(reference=w352, error in=w351, "channel"=w346, "length"=w348) -> (reference out=w345:refnum<k7>, error out=w344:errorcluster)  [unwired: 1 in, 3 out]
                    n132 = invoke class="IBSA" method="SetRecordLengthMode"(reference=w345, error in=w344, "channel"=w346, "mode"=1) -> (reference out=w342:refnum<k7>, error out=w343:errorcluster)  [unwired: 1 in, 3 out]
                  }
                  frame "Signal gain (dB)" {
                    n133 = Decimal String To Number(string=w358) -> (number=w353:i32)  [unwired: 3 out]
                    n134 = In Range and Coerce(upper limit=30, x=w353, lower limit=0) -> (coerced(x)=w354:i32)  [unwired: 1 out]
                    n135 = invoke class="IBSA" method="SetSignalGain"(reference=w362, error in=w359, "channel"=w363, "gain"=w354) -> (reference out=w361:refnum<k7>, error out=w360:errorcluster)  [unwired: 1 in, 3 out]
                  }
                  frame "High Voltage" {
                    n136 = Decimal String To Number(string=w365) -> (number=w366:i32)  [unwired: 3 out]
                    n137 = invoke class="IBSA" method="SetHighVoltage"(reference=w370, error in=w367, "channel"=w371, "volt"=w366) -> (reference out=w369:refnum<k7>, error out=w368:errorcluster)  [unwired: 1 in, 3 out]
                  }
                  frame "Component" {
                    n138 = invoke class="IBSA" method="SetAnodeCurrentLimit"(reference=w373, error in=w372, "channel"=w377, "limit"=1500) -> (reference out=w374:refnum<k7>, error out=w375:errorcluster)  [unwired: 1 in, 3 out]
                    n139 = Bundle By Name(cluster=w380, "Vel Comp"=w379) -> (w378:T6)
                  }
                  frame "Level_Validation_Ratio" {
                    n140 = Decimal String To Number(string=w384) -> (number=w383:i32)  [unwired: 3 out]
                    n141 = invoke class="IBSA" method="SetLevelValidationRatio"(reference=w388, error in=w387, "channel"=w386, "ratio"=w383) -> (reference out=w381:refnum<k7>, error out=w382:errorcluster)  [unwired: 1 in, 3 out]
                  }
                  frame "Burst_Detector_Signal_to_Noise_Ratio" {
                    n142 = Decimal String To Number(string=w392) -> (number=w391:i32)  [unwired: 3 out]
                    n143 = invoke class="IBSA" method="SetBurstDetectorSNR"(reference=w396, error in=w395, "channel"=w394, "snr"=w391) -> (reference out=w389:refnum<k7>, error out=w390:errorcluster)  [unwired: 1 in, 3 out]
                  }
                  frame "Multiply Velocity by -1" {
                    n144 = Equal?(x="TRUE", y=w401) -> (x = y?=w399:bool)
                    n145 = Bundle By Name(cluster=w403, "Multiply Velocity by -1"=w399) -> (w402:T6)
                  }
                  frame "Bandwidth" {
                    n146 = call "String_2_Number.vi"("Value"=w408) -> ("Numeric"=w407:dbl)
                    n147 = Unbundle By Name(w406) -> ("Optics Conversion Factor"=w405:dbl)
                    n148 = Divide(x=w407, y=w405) -> (x/y=w404:dbl)
                    n149 = invoke class="IBSA" method="SetBandwidth"(reference=w412, error in=w409, "channel"=w413, "bandwidth"=w404) -> (reference out=w411:refnum<k7>, error out=w410:errorcluster)  [unwired: 1 in, 3 out]
                  }
                  frame "Centre frequency" {
                    n150 = call "String_2_Number.vi"("Value"=w418) -> ("Numeric"=w417:dbl)
                    n151 = Unbundle By Name(w416) -> ("Optics Conversion Factor"=w415:dbl)
                    n152 = Divide(x=w417, y=w415) -> (x/y=w414:dbl)
                    n153 = invoke class="IBSA" method="SetCenterFreq"(reference=w422, error in=w419, "channel"=w423, "freq"=w414) -> (reference out=w421:refnum<k7>, error out=w420:errorcluster)  [unwired: 1 in, 3 out]
                  }
                }
              }
              frame "Char not in string" {
              }
            }
          }
        }
      }
      frame "Read Values back from BSA" {
        n154 = local read "Setup String to read"() -> (w427:string)
        n155 = for {
          tunnel: w427 -> [w448]
          tunnel: w438 -> [w447]
          tunnel: [w446] -> w437
          shift-right: [w443] -> w435
          shift-left: w436 -> [w444]
          tunnel: w433 -> [w445]
          tunnel: w434 -> [w442] mode=indexing
          tunnel: [w441] -> w432 mode=indexing
          i -> [w440]
          n156 = for {
            tunnel: w440 -> [w457]
            tunnel: w448 -> [w451]
            tunnel: w447 -> [w456]
            tunnel: [w455] -> w446
            tunnel: w445 -> [w454] mode=indexing
            shift-right: [w452] -> w443
            shift-left: w444 -> [w453]
            shift-right: [w449] -> w441
            shift-left: w442 -> [w450]
            n157 = case shown="\"Centre frequency\"" w454 {
              tunnel: w457 -> [_ w477 w489 w497 w506 w515 w523 _ _ w537 w552]
              tunnel: w456 -> [w465 w476 w488 w496 w505 w514 w522 w525 w528 w541 w556]
              tunnel: [w465 w475 w487 w495 w504 w513 w521 w525 w528 w540 w555] -> w455
              tunnel: [w464 w474 w486 w494 w503 w512 w520 w526 w529 w539 w554] -> w452
              tunnel: w453 -> [w464 w473 w485 w493 w502 w511 w519 w526 w529 w538 w553]
              tunnel: w454 -> [w463 _ _ _ _ _ _ _ _ _ _]
              tunnel: w450 -> [w458 w472 w484 w491 w501 w510 w518 w524 w527 w532 w548]
              tunnel: w451 -> [_ _ _ _ _ _ _ _ _ _ _]
              tunnel: [w458 w471 w483 w490 w500 w509 w517 w524 w527 w530 w548] -> w449
              frame "No Match", Default {
                n158 = Concatenate Strings(w463, " has not been matched" ("string")) -> (w461:string)
                n159 = One Button Dialog(message=w461, button name ("OK")="Stop") -> (true=w459:bool)
                n160 = Stop(stop? (T)=w459) -> ()
              }
              frame "Record length" {
                n161 = local read "Record Length"() -> (w468:dbl[])
                n162 = invoke class="IBSA" method="GetRecordLength"(reference=w476, error in=w473, "channel"=w477) -> (reference out=w475:refnum<k7>, error out=w474:errorcluster, "GetRecordLength"=w467:i32)  [unwired: 1 in, 1 out]
                n163 = Subtract(x=w468, y=w467) -> (x-y=w470:dbl[])
                n164 = Absolute Value(x=w470) -> (abs(x)=w469:dbl[])
                n165 = Array Max & Min(array=w469) -> (min index (indices)=w466:i32)  [unwired: 3 out]
                n166 = Bundle By Name(cluster=w472, "Min Record length"=w466) -> (w471:T6)
              }
              frame "Max Record length" {
                n167 = local read "Record Length"() -> (w480:dbl[])
                n168 = invoke class="IBSA" method="GetMaxRecordLength"(reference=w488, error in=w485, "channel"=w489) -> (reference out=w487:refnum<k7>, error out=w486:errorcluster, "GetMaxRecordLength"=w479:i32)  [unwired: 1 in, 1 out]
                n169 = Subtract(x=w480, y=w479) -> (x-y=w482:dbl[])
                n170 = Absolute Value(x=w482) -> (abs(x)=w481:dbl[])
                n171 = Array Max & Min(array=w481) -> (min index (indices)=w478:i32)  [unwired: 3 out]
                n172 = Bundle By Name(cluster=w484, "Max Record length"=w478) -> (w483:T6)
              }
              frame "Signal gain (dB)" {
                n173 = invoke class="IBSA" method="GetSignalGain"(reference=w496, error in=w493, "channel"=w497) -> (reference out=w495:refnum<k7>, error out=w494:errorcluster, "GetSignalGain"=w492:i32)  [unwired: 1 in, 1 out]
                n174 = Bundle By Name(cluster=w491, "Signal gain (dB)"=w492) -> (w490:T6)
              }
              frame "Burst_Detector_Signal_to_Noise_Ratio" {
                n175 = invoke class="IBSA" method="GetBurstDetectorSNR"(reference=w505, error in=w502, "channel"=w506) -> (reference out=w504:refnum<k7>, error out=w503:errorcluster, "GetBurstDetectorSNR"=w498:i32)  [unwired: 1 in, 1 out]
                n176 = Number To Decimal String(number=w498) -> (decimal integer string=w499:string)  [unwired: 1 out]
                n177 = Bundle By Name(cluster=w501, "Signal to Noise Ratio"=w499) -> (w500:T6)
              }
              frame "Level_Validation_Ratio" {
                n178 = invoke class="IBSA" method="GetLevelValidationRatio"(reference=w514, error in=w511, "channel"=w515) -> (reference out=w513:refnum<k7>, error out=w512:errorcluster, "GetLevelValidationRatio"=w507:i32)  [unwired: 1 in, 1 out]
                n179 = Number To Decimal String(number=w507) -> (decimal integer string=w508:string)  [unwired: 1 out]
                n180 = Bundle By Name(cluster=w510, "Validation Ratio"=w508) -> (w509:T6)
              }
              frame "High Voltage" {
                n181 = invoke class="IBSA" method="GetHighVoltage"(reference=w522, error in=w519, "channel"=w523) -> (reference out=w521:refnum<k7>, error out=w520:errorcluster, "GetHighVoltage"=w516:i32)  [unwired: 1 in, 1 out]
                n182 = Bundle By Name(cluster=w518, "High voltage"=w516) -> (w517:T6)
              }
              frame "Component" {
              }
              frame "Multiply Velocity by -1" {
              }
              frame "Bandwidth" {
                n183 = local read "Bandwidth Array Hz"() -> (w534:dbl[])
                n184 = invoke class="IBSA" method="GetBandwidth"(reference=w541, error in=w538, "channel"=w537) -> (reference out=w540:refnum<k7>, error out=w539:errorcluster, "GetBandwidth"=w531:sgl)  [unwired: 1 in, 1 out]
                n185 = Bundle By Name(cluster=w532, "Bandwidth Hz"=w531) -> (w530:T6)
                n186 = Subtract(x=w534, y=w531) -> (x-y=w536:dbl[])
                n187 = Absolute Value(x=w536) -> (abs(x)=w535:dbl[])
                n188 = Array Max & Min(array=w535) -> (min index (indices)=w533:i32)  [unwired: 3 out]
                n189 = case shown="1" w537 {
                  tunnel: w533 -> [w542 w543]
                  frame 0, Default {
                    n190 = local write "Bandwidth 0"(w542) -> ()
                  }
                  frame 1 {
                    n191 = local write "Bandwidth 1"(w543) -> ()
                  }
                }
              }
              frame "Centre frequency" {
                n192 = local read "C Array"() -> (w547:dbl[])
                n193 = Unbundle By Name(w548) -> ("Bandwidth Hz"=w545:dbl)
                n194 = invoke class="IBSA" method="GetCenterFreq"(reference=w556, error in=w553, "channel"=w552) -> (reference out=w555:refnum<k7>, error out=w554:errorcluster, "GetCenterFreq"=w546:sgl)  [unwired: 1 in, 1 out]
                n195 = Divide(x=w546, y=w545) -> (x/y=w544:dbl)
                n196 = Subtract(x=w547, y=w544) -> (x-y=w551:dbl[])
                n197 = Absolute Value(x=w551) -> (abs(x)=w550:dbl[])
                n198 = Array Max & Min(array=w550) -> (min index (indices)=w549:i32)  [unwired: 3 out]
                n199 = case shown="1" w552 {
                  tunnel: w549 -> [w557 w558]
                  frame 0, Default {
                    n200 = local write "Centre frequency 0"(w557) -> ()
                  }
                  frame 1 {
                    n201 = local write "Centre frequency 1"(w558) -> ()
                  }
                }
              }
            }
          }
        }
        n202 = local read "Final read?"() -> (w431:bool)
        n203 = local write "Setup Array"(w432) -> ()
        n204 = Select(t="Update Globals", s=w431, f="Loop") -> (s? t:f=w428:string)
      }
      frame "Loop" {
        n205 = local read "Focal Lengths Cluster"() -> (w559:cluster{"Focal Lengths":string[]}[])
        n206 = local read "Bandwidth Array Hz"() -> (w574:dbl[])
        n207 = local read "C Array"() -> (w573:dbl[])
        n208 = Wait Until Next ms Multiple(millisecond multiple=u32 300) -> ()  [unwired: 1 out]
        n209 = for {
          tunnel: w574 -> [w582]
          tunnel: w573 -> [w579]
          tunnel: [w581] -> w571 mode=indexing
          tunnel: "Setup Array" -> [w578] mode=indexing
          tunnel: w559 -> [w577]
          i -> [w580]
          # "cf"
          # "BS"
          # "FL"
          # "WL"
          n210 = stacked-sequence {
            seq-local: [w584 _ _ _ _ _] -> [_ _ _ w613 _ w683]
            seq-local: [_ w596 _ _ _ _] -> [_ _ _ w621 _ w680]
            seq-local: [_ _ w605 _ _ _] -> [_ _ _ w622 _ w679]
            seq-local: [_ _ _ w618 _ _] -> [_ _ _ _ w626 w682]
            seq-local: [_ _ _ _ w625 _] -> [_ _ _ _ _ w684]
            seq-local: [w583 _ _ _ _ _] -> [_ _ _ _ _ w677]
            tunnel: w582 -> [_ _ _ w617 w652 _]
            tunnel: [_ _ _ _ _ w678] -> w581
            tunnel: w580 -> [_ w598 _ w619 w649 w681]
            tunnel: w579 -> [_ _ _ _ w637 _]
            tunnel: w578 -> [w586 w595 w609 _ w627 _]
            tunnel: w577 -> [_ w591 _ _ _ _]
            frame #0 {
              n211 = Unbundle By Name(w586) -> ("Beams Colour"=w585:u16)
              n212 = case shown="0, Default" w585 {
                tunnel: [w587 w589] -> w584
                tunnel: [u32 6618880 u32 3381759] -> w583
                frame 0, Default {
                  n213 = local read "Green Wavelength"() -> (w587:dbl)
                }
                frame 1 {
                  n214 = local read "Blue Wavelength"() -> (w589:dbl)
                }
              }
            }
            frame #1 {
              n215 = Unbundle By Name(w595) -> ("Probe Type"=w594:u16)
              n216 = Index Array(array=w591, index=w594) -> (element=w593:cluster{"Focal Lengths":string[]})
              n217 = Unbundle By Name(w593) -> ("Focal Lengths"=w592:string[])
              n218 = case shown="1" w598 {
                tunnel: [w600 w604] -> w597
                tunnel: w592 -> [w599 w603]
                frame 0, Default {
                  n219 = property on="Focal Length 0" class="Ring (strict)"("Strings []"=w599) -> ()  [unwired: 2 in, 2 out]
                  n220 = Index Array(array=w599, index="Focal Length 0") -> (element=w600:string)
                }
                frame 1 {
                  n221 = property on="Focal Length 1" class="Ring (strict)"("Strings []"=w603) -> ()  [unwired: 2 in, 2 out]
                  n222 = Index Array(array=w603, index="Focal Length 1") -> (element=w604:string)
                }
              }
              n223 = Fract/Exp String To Number(string=w597) -> (number=w596:dbl)  [unwired: 3 in, 1 out]
            }
            frame #2 {
              n224 = Unbundle By Name(w609) -> ("Fibre Colour"=w608:u16, "Probe Type"=w606:u16)
              n225 = case shown="0, Default" w608 {
                tunnel: [w610 w611] -> w607
                frame 0, Default {
                  n226 = local read "Green Fibre Separation"() -> (w610:dbl[])
                }
                frame 1 {
                  n227 = local read "Blue Fibre Separation"() -> (w611:dbl[])
                }
              }
              n228 = Index Array(array=w607, index=w606) -> (element=w605:dbl)
            }
            frame #3 {
              n229 = Multiply(x=w613, y=1e-09) -> (x*y=w612:dbl)
              n230 = formula code="cf = 0.5 * lam/(sin(atan(0.5 * bs / fl)));"("bs"=w622, "fl"=w621, "lam"=w612) -> ("cf"=w618:dbl)
              n231 = Multiply(x=w618, y=w617) -> (x*y=w616:dbl[])
              n232 = Number To Fractional String(number=w616, precision (6)=i16 3) -> (F-format string=w615:string[])  [unwired: 2 out]
              n233 = case shown="1" w619 {
                tunnel: w615 -> [w623 w624]
                frame 0, Default {
                  n234 = property on="Bandwidth 0" class="Ring (strict)"("Strings []"=w623) -> ()  [unwired: 2 in, 2 out]
                }
                frame 1 {
                  n235 = property on="Bandwidth 1" class="Ring (strict)"("Strings []"=w624) -> ()  [unwired: 2 in, 2 out]
                }
              }
            }
            frame #4 {
              n236 = Unbundle By Name(w627) -> ("Max Record length"=w642:u16, "Min Record length"=w644:u16, "Multiply Velocity by -1"=w636:bool)
              n237 = case shown="0, Default" w649 {
                tunnel: ["Bandwidth 0" "Bandwidth 1"] -> w653
                tunnel: ["Centre frequency 0" "Centre frequency 1"] -> w651
                frame 0, Default {
                }
                frame 1 {
                }
              }
              n238 = Greater Or Equal?(x=w642, y=w644) -> (x >= y?=w643:bool)
              n239 = case shown="False" w643 {
                tunnel: w627 -> [w665 w666]
                tunnel: w642 -> [w664 _]
                tunnel: [w663 w666] -> w641
                frame False {
                  n240 = Bundle By Name(cluster=w665, "Min Record length"=w664) -> (w663:T6)
                }
                frame True {
                }
              }
              n241 = Index Array(array=w652, index=w653) -> (element=w648:dbl)
              n242 = Multiply(x=w626, y=w648) -> (x*y=w646:dbl)
              n243 = Multiply(x=w637, y=w646) -> (x*y=w633:dbl[])
              n244 = Index Array(array=w633, index=w651) -> (element=w638:dbl)
              n245 = Divide(x=w646, y=2.0) -> (x/y=w639:dbl)
              n246 = Negate(x=w639) -> (-x=w640:dbl)
              n247 = Add(x=w640, y=w638) -> (x+y=w634:dbl)
              n248 = Add(x=w639, y=w638) -> (x+y=w635:dbl)
              n249 = case shown="False" w636 {
                tunnel: [w654 w660] -> w628
                tunnel: w635 -> [w654 w662]
                tunnel: [w656 w659] -> w629
                tunnel: w634 -> [w656 w661]
                tunnel: w633 -> [w655 w658]
                tunnel: [w655 w657] -> w632
                frame False {
                }
                frame True {
                  n250 = Negate(x=w661) -> (-x=w659:dbl)
                  n251 = Negate(x=w662) -> (-x=w660:dbl)
                  n252 = Negate(x=w658) -> (-x=w657:dbl[])
                }
              }
              n253 = Max & Min(x=w629, y=w628) -> (max(x,y)=w630:dbl, min(x,y)=w631:dbl)
              n254 = Bundle By Name(cluster=w641, "Max Velocity"=w630, "Min Velocity"=w631) -> (w625:T6)
              n255 = Number To Fractional String(number=w632, precision (6)=i16 3) -> (F-format string=w645:string[])  [unwired: 2 out]
              n256 = case shown="0, Default" w649 {
                tunnel: w646 -> [w669 w672]
                tunnel: w638 -> [w668 w671]
                tunnel: w645 -> [w667 w670]
                frame 0, Default {
                  n257 = global write "LDA_meas_global_1.vi" "Bandwidth BSA1"(w669) -> ()
                  n258 = global write "LDA_meas_global_1.vi" "Centre Freq BSA1"(w668) -> ()
                  n259 = property on="Centre frequency 0" class="Ring (strict)"("Strings []"=w667) -> ()  [unwired: 2 in, 2 out]
                }
                frame 1 {
                  n260 = global write "LDA_meas_global_2.vi" "Centre Freq BSA2"(w671) -> ()
                  n261 = global write "LDA_meas_global_2.vi" "Bandwidth BSA2"(w672) -> ()
                  n262 = property on="Centre frequency 1" class="Ring (strict)"("Strings []"=w670) -> ()  [unwired: 2 in, 2 out]
                }
              }
            }
            frame #5 {
              n263 = case shown="1" w681 {
                tunnel: w680 -> [w686 w688]
                tunnel: w679 -> [w685 w687]
                frame 0, Default {
                  n264 = global write "LDA_meas_global_1.vi" "Focal Length (mm)"(w686) -> ()
                  n265 = global write "LDA_meas_global_1.vi" "Beam Separation (mm)"(w685) -> ()
                }
                frame 1 {
                  n266 = global write "LDA_meas_global_2.vi" "Beam Separation 2 (mm)"(w687) -> ()
                  n267 = global write "LDA_meas_global_2.vi" "Focal Length 2 (mm)"(w688) -> ()
                }
              }
              n268 = Bundle By Name(cluster=w684, "Wavelength (nm)"=w683, "Optics Conversion Factor"=w682, "COLOUR"=w677) -> (w678:T6)
            }
          }
        }
        n269 = Not Equal?(x=w571, y="Setup Array") -> (x != y?=w572:bool)
        n270 = case shown="True" w572 {
          tunnel: w571 -> [_ w576]
          frame False {
          }
          frame True {
            n271 = local write "Setup Array"(w576) -> ()
          }
        }
        n272 = Compound Arithmetic op=AND(invert "Run LDA Diagnostic", invert "OK", w562) -> (w566:bool)
        n273 = Select(t="Loop", s=w566, f="Check Vel Component") -> (s? t:f=w565:string)
        "Run LDA Diagnostic Out" <- "Run LDA Diagnostic"
      }
      frame "Check Vel Component" {
        n274 = for {
          tunnel: w689 -> [w705] mode=indexing
          shift-right: [w703] -> _
          shift-left: "" -> [w704]
          tunnel: [w700] -> w694 mode=indexing
          n275 = Unbundle By Name(w705) -> ("Vel Comp"=w703:string)
          n276 = Empty String/Path?(string/path=w703) -> (empty?=w702:bool)
          n277 = Not Equal?(x=w703, y=w704) -> (x != y?=w701:bool)
          n278 = Compound Arithmetic op=AND(invert w702, w701) -> (w700:bool)
        }
        n279 = And Array Elements(Boolean array=w694) -> (logical AND=w693:bool)
        n280 = case shown="False" w693 {
          tunnel: ["Loop" "Write Setup to BSA" ("f")] -> w690
          frame False {
            n281 = One Button Dialog(message="The \"Vel Comp\" should not be blank or the same") -> ()  [unwired: 1 in, 1 out]
          }
          frame True {
          }
        }
      }
      frame "Write Setup to BSA" {
        n282 = local read "Setup String to read"() -> (w706:string)
        n283 = for {
          tunnel: w706 -> [w725]
          tunnel: w714 -> [w724]
          tunnel: [w723] -> w713
          shift-right: [w720] -> w711
          shift-left: w712 -> [w721]
          tunnel: w708 -> [w722]
          tunnel: w710 -> [w718] mode=indexing
          tunnel: [w717] -> w709 mode=indexing
          i -> [w719]
          n284 = for {
            tunnel: w719 -> [w734]
            tunnel: w725 -> [w728]
            tunnel: w724 -> [w733]
            tunnel: [w732] -> w723
            tunnel: w722 -> [w731] mode=indexing
            shift-right: [w729] -> w720
            shift-left: w721 -> [w730]
            shift-right: [w726] -> w717
            shift-left: w718 -> [w727]
            n285 = case shown="\"Burst_Detector_Signal_to_Noise_Ratio\"" w731 {
              tunnel: w734 -> [_ w751 w760 w767 w774 w782 w790 _ _ w802 w814]
              tunnel: w733 -> [w742 w750 w759 w766 w773 w781 w789 w792 w795 w806 w819]
              tunnel: [w742 w749 w758 w765 w772 w780 w788 w792 w795 w805 w818] -> w732
              tunnel: [w741 w748 w757 w764 w771 w779 w787 w793 w796 w804 w817] -> w729
              tunnel: w730 -> [w741 w747 w756 w763 w770 w778 w786 w793 w796 w803 w816]
              tunnel: w731 -> [w740 _ _ _ _ _ _ _ _ _ _]
              tunnel: w727 -> [w735 w746 w755 w762 w769 w777 w785 w791 w794 w799 w815]
              tunnel: w728 -> [_ _ _ _ _ _ _ _ _ _ _]
              tunnel: [w735 w746 w755 w762 w769 w777 w785 w791 w794 w798 w815] -> w726
              frame "No Match", Default {
                n286 = Concatenate Strings(w740, " has not been matched" ("string")) -> (w738:string)
                n287 = One Button Dialog(message=w738, button name ("OK")="Stop") -> (true=w736:bool)
                n288 = Stop(stop? (T)=w736) -> ()
              }
              frame "Record length" {
                n289 = Unbundle By Name(w746) -> ("Min Record length"=w744:u16)
                n290 = local read "Record Length"() -> (w745:dbl[])
                n291 = Index Array(array=w745, index=w744) -> (element=w743:dbl)
                n292 = invoke class="IBSA" method="SetRecordLength"(reference=w750, error in=w747, "channel"=w751, "length"=w743) -> (reference out=w749:refnum<k7>, error out=w748:errorcluster)  [unwired: 1 in, 3 out]
              }
              frame "Max Record length" {
                n293 = Unbundle By Name(w755) -> ("Max Record length"=w753:u16)
                n294 = local read "Record Length"() -> (w754:dbl[])
                n295 = Index Array(array=w754, index=w753) -> (element=w752:dbl)
                n296 = invoke class="IBSA" method="SetMaxRecordLength"(reference=w759, error in=w756, "channel"=w760, "length"=w752) -> (reference out=w758:refnum<k7>, error out=w757:errorcluster)  [unwired: 1 in, 3 out]
              }
              frame "Signal gain (dB)" {
                n297 = Unbundle By Name(w762) -> ("Signal gain (dB)"=w761:i16)
                n298 = invoke class="IBSA" method="SetSignalGain"(reference=w766, error in=w763, "channel"=w767, "gain"=w761) -> (reference out=w765:refnum<k7>, error out=w764:errorcluster)  [unwired: 1 in, 3 out]
              }
              frame "High Voltage" {
                n299 = Unbundle By Name(w769) -> ("High voltage"=w768:i16)
                n300 = invoke class="IBSA" method="SetHighVoltage"(reference=w773, error in=w770, "channel"=w774, "volt"=w768) -> (reference out=w772:refnum<k7>, error out=w771:errorcluster)  [unwired: 1 in, 3 out]
              }
              frame "Level_Validation_Ratio" {
                n301 = Unbundle By Name(w777) -> ("Validation Ratio"=w776:string)
                n302 = Decimal String To Number(string=w776) -> (number=w775:i32)  [unwired: 3 out]
                n303 = invoke class="IBSA" method="SetLevelValidationRatio"(reference=w781, error in=w778, "channel"=w782, "ratio"=w775) -> (reference out=w780:refnum<k7>, error out=w779:errorcluster)  [unwired: 1 in, 3 out]
              }
              frame "Burst_Detector_Signal_to_Noise_Ratio" {
                n304 = Unbundle By Name(w785) -> ("Signal to Noise Ratio"=w784:string)
                n305 = Decimal String To Number(string=w784) -> (number=w783:i32)  [unwired: 3 out]
                n306 = invoke class="IBSA" method="SetBurstDetectorSNR"(reference=w789, error in=w786, "channel"=w790, "snr"=w783) -> (reference out=w788:refnum<k7>, error out=w787:errorcluster)  [unwired: 1 in, 3 out]
              }
              frame "Component" {
              }
              frame "Multiply Velocity by -1" {
              }
              frame "Bandwidth" {
                n307 = case shown="1" w802 {
                  tunnel: [w807 w808] -> w801
                  frame 0, Default {
                    n308 = local read "Bandwidth 0"() -> (w807:u16)
                  }
                  frame 1 {
                    n309 = local read "Bandwidth 1"() -> (w808:u16)
                  }
                }
                n310 = local read "Bandwidth Array Hz"() -> (w800:dbl[])
                n311 = Index Array(array=w800, index=w801) -> (element=w797:dbl)
                n312 = Bundle By Name(cluster=w799, "Bandwidth Hz"=w797) -> (w798:T6)
                n313 = invoke class="IBSA" method="SetBandwidth"(reference=w806, error in=w803, "channel"=w802, "bandwidth"=w797) -> (reference out=w805:refnum<k7>, error out=w804:errorcluster)  [unwired: 1 in, 3 out]
              }
              frame "Centre frequency" {
                n314 = case shown="1" w814 {
                  tunnel: [w820 w821] -> w813
                  frame 0, Default {
                    n315 = local read "Centre frequency 0"() -> (w820:u16)
                  }
                  frame 1 {
                    n316 = local read "Centre frequency 1"() -> (w821:u16)
                  }
                }
                n317 = Unbundle By Name(w815) -> ("Bandwidth Hz"=w810:dbl)
                n318 = local read "C Array"() -> (w812:dbl[])
                n319 = Index Array(array=w812, index=w813) -> (element=w811:dbl)
                n320 = Multiply(x=w810, y=w811) -> (x*y=w809:dbl)
                n321 = invoke class="IBSA" method="SetCenterFreq"(reference=w819, error in=w816, "channel"=w814, "freq"=w809) -> (reference out=w818:refnum<k7>, error out=w817:errorcluster)  [unwired: 1 in, 3 out]
              }
            }
          }
        }
        n322 = local write "Final read?"(TRUE ("Boolean")) -> ()
      }
      frame "Error" {
        n323 = call "EnFlo_Error_Handler.vi"("error in (no error)"=w825, "Dialog Box (T)"=FALSE) -> ()  [unwired: 1 in, 3 out]
      }
      frame "Update Globals" {
        n324 = local read "Probe Options"() -> (w831:string[])
        n325 = for {
          tunnel: w835 -> [w840] mode=indexing
          tunnel: w831 -> [w838]
          tunnel: w829 -> [w837]
          i -> [w839]
          n326 = stacked-sequence {
            seq-local: [w854 _] -> [_ w873]
            tunnel: w840 -> [w868 w887]
            tunnel: w839 -> [w863 w874]
            tunnel: w838 -> [w844 _]
            tunnel: w837 -> [w842 w871]
            frame #0 {
              n327 = Increment(x=w863) -> (x+1=w866:i32)
              n328 = Unbundle By Name(w868) -> ("Signal to Noise Ratio"=w860:string, "Validation Ratio"=w858:string, "Probe Type"=w851:u16, "Fibre Colour"=w843:u16)
              n329 = Number To Decimal String(number=w866) -> (decimal integer string=w864:string)  [unwired: 1 out]
              n330 = Index Array(array=w842, index=w843) -> (element=w841:string)
              n331 = Concatenate Strings("BSA ", w864, " ") -> (w847:string)
              n332 = Concatenate Strings(w847, "Burst_Detector_Signal_to_Noise_Ratio" ("Pre Setup String")) -> (w861:string)
              n333 = Concatenate Strings(w847, "Level_Validation_Ratio" ("Pre Setup String")) -> (w859:string)
              n334 = Concatenate Strings(w847, "Probe_Type" ("Pre Setup String")) -> (w852:string)
              n335 = Index Array(array=w844, index=w851) -> (element=w850:string)
              n336 = Concatenate Strings(w847, "Fibre_Colour" ("string")) -> (w848:string)
              n337 = call "Characters_to_string.vi"("Characters to write"=w860, "Label for characters"=w861) -> ("Output string"=w855:string)
              n338 = call "Characters_to_string.vi"("Characters to write"=w858, "Label for characters"=w859) -> ("Output string"=w856:string)
              n339 = call "Characters_to_string.vi"("Characters to write"=w841, "Label for characters"=w848) -> ("Output string"=w845:string)
              n340 = call "Characters_to_string.vi"("Characters to write"=w850, "Label for characters"=w852) -> ("Output string"=w849:string)
              n341 = Concatenate Strings(w855, w856, w849, w845) -> (w854:string)
            }
            frame #1 {
              n342 = Unbundle By Name(w887) -> ("Max Record length"=w879:u16, "Min Record length"=w881:u16, "Vel Comp"=w886:string, "Signal gain (dB)"=w885:i16, "High voltage"=w884:i16, "Max Velocity"=w883:dbl, "Min Velocity"=w882:dbl, "Optics Conversion Factor"=w876:dbl, "Multiply Velocity by -1"=w875:bool, "Wavelength (nm)"=w872:dbl, "Beams Colour"=w869:u16)
              n343 = local read "Record Length"() -> (w878:dbl[])
              n344 = Index Array(array=w871, index=w869) -> (element=w870:string)
              n345 = Index Array(array=w878, index=w879) -> (element=w877:dbl)
              n346 = Index Array(array=w878, index=w881) -> (element=w880:dbl)
              n347 = case shown="1" w874 {
                tunnel: w880 -> [w899 w911]
                tunnel: w886 -> [w898 w905]
                tunnel: w885 -> [w897 w906]
                tunnel: w884 -> [w896 w907]
                tunnel: w883 -> [w895 w908]
                tunnel: w882 -> [w894 w909]
                tunnel: w876 -> [w893 w910]
                tunnel: w877 -> [w892 w904]
                tunnel: w875 -> [w891 w903]
                tunnel: w873 -> [w890 w902]
                tunnel: w872 -> [w889 w901]
                tunnel: w870 -> [w888 w900]
                frame 0, Default {
                  n348 = global write "LDA_meas_global_1.vi" "Max Record length BSA1"(w892) -> ()
                  n349 = global write "LDA_meas_global_1.vi" "Optic Calib factor BSA1"(w893) -> ()
                  n350 = global write "LDA_meas_global_1.vi" "Vel Comp BSA1"(w898) -> ()
                  n351 = global write "LDA_meas_global_1.vi" "Additional BSA1 Setup"(w890) -> ()
                  n352 = global write "LDA_meas_global_1.vi" "Multiply Velocity by -1"(w891) -> ()
                  n353 = global write "LDA_meas_global_1.vi" "Record length BSA1"(w899) -> ()
                  n354 = global write "LDA_meas_global_1.vi" "Wavelength 1 (nm)"(w889) -> ()
                  n355 = global write "LDA_meas_global_1.vi" "Signal gain BSA1"(w897) -> ()
                  n356 = global write "LDA_meas_global_1.vi" "Beams Colour 1"(w888) -> ()
                  n357 = global write "LDA_meas_global_1.vi" "High Volt BSA1"(w896) -> ()
                  n358 = global write "LDA_meas_global_1.vi" "Min Vel BSA1"(w894) -> ()
                  n359 = global write "LDA_meas_global_1.vi" "Max Vel BSA1"(w895) -> ()
                }
                frame 1 {
                  n360 = global write "LDA_meas_global_2.vi" "Max Record length BSA2"(w904) -> ()
                  n361 = global write "LDA_meas_global_2.vi" "Optic Calib factor BSA2"(w910) -> ()
                  n362 = global write "LDA_meas_global_2.vi" "Additional BSA2 Setup"(w902) -> ()
                  n363 = global write "LDA_meas_global_2.vi" "Multiply Velocity by -1"(w903) -> ()
                  n364 = global write "LDA_meas_global_2.vi" "Wavelength 2 (nm)"(w901) -> ()
                  n365 = global write "LDA_meas_global_2.vi" "Record length BSA2"(w911) -> ()
                  n366 = global write "LDA_meas_global_2.vi" "Beams Colour 2"(w900) -> ()
                  n367 = global write "LDA_meas_global_2.vi" "Signal gain BSA2"(w906) -> ()
                  n368 = global write "LDA_meas_global_2.vi" "Vel Comp BSA2"(w905) -> ()
                  n369 = global write "LDA_meas_global_2.vi" "High Volt BSA2"(w907) -> ()
                  n370 = global write "LDA_meas_global_2.vi" "Max Vel BSA2"(w908) -> ()
                  n371 = global write "LDA_meas_global_2.vi" "Min Vel BSA2"(w909) -> ()
                }
              }
            }
          }
        }
        n372 = global write "LDA_meas_global_1.vi" "Non-coincident"("Non-coincident") -> ()
      }
      frame "Write LDA Probe File" {
        n373 = stacked-sequence {
          seq-local: [_ w963 _ _] -> [_ _ w975 _]
          seq-local: [w935 _ _ _] -> [_ _ w976 _]
          tunnel: [_ _ _ FALSE] -> w931
          tunnel: w930 -> [_ _ _ w995]
          tunnel: [_ _ _ w995] -> w929
          tunnel: [_ _ _ "End"] -> w928
          tunnel: w927 -> [_ _ _ w993]
          tunnel: [_ _ _ w993] -> w926
          tunnel: w925 -> [_ _ _ w992]
          tunnel: [_ _ _ w992] -> w924
          tunnel: w923 -> [_ w968 _ _]
          tunnel: w922 -> [_ w967 _ _]
          tunnel: w921 -> [_ w966 _ _]
          tunnel: w920 -> [_ w965 _ _]
          tunnel: w919 -> [w943 _ _ _]
          tunnel: w918 -> [w944 _ _ _]
          tunnel: w917 -> [w942 _ _ _]
          tunnel: w916 -> [w940 _ _ _]
          tunnel: w915 -> [w934 _ _ _]
          tunnel: w914 -> [_ _ w974 _]
          tunnel: w913 -> [_ w956 _ _]
          tunnel: w912 -> [_ w955 _ _]
          frame #0 {
            n374 = global write "LDA_meas_global_1.vi" "Using 45 Degree Mirror?"("45 Degree Mirror") -> ()
            n375 = Index Array(array=w934, index="Beam Alignment") -> (element=w941:string)
            n376 = call "BSA_Type_String.vi"("BSA Type"="BSA Type") -> ("BSA String Out"=w945:string)  [unwired: 1 in, 1 out]
            n377 = Select(t="TRUE", s="45 Degree Mirror", f="FALSE") -> (s? t:f=w950:string)
            n378 = call "Characters_to_string.vi"("Characters to write"="BSA IP Number", "Label for characters"=w940) -> ("Output string"=w939:string)
            n379 = call "Characters_to_string.vi"("Characters to write"=w945, "Label for characters"=w944) -> ("Output string"=w936:string)
            n380 = call "Characters_to_string.vi"("Characters to write"=w950, "Label for characters"=w943) -> ("Output string"=w937:string)
            n381 = call "Characters_to_string.vi"("Characters to write"=w941, "Label for characters"=w942) -> ("Output string"=w938:string)
            n382 = global write "LDA_meas_global_1.vi" "BSA IP Number"("BSA IP Number") -> ()
            n383 = Concatenate Strings(w939, w938, w937, w936) -> (w935:string)
          }
          frame #1 {
            w957 = "3" ("precision")
            w962 = "\r\n"
            w969 = "0" ("precision")
            n384 = Unbundle By Name("Warn if Power below (mW)") -> ("Green Unshifted"=w961:i32, "Green Shifted"=w960:i32, "Blue Unshifted"=w959:i32, "Blue Shifted"=w958:i32)
            n385 = local read "Green Wavelength"() -> (w954:dbl)
            n386 = local read "Blue Wavelength"() -> (w953:dbl)
            n387 = call "Value_to_string.vi"("precision"=w957, "Value"=w954, "Label for value"=w956) -> ("Output string"=w952:string)
            n388 = call "Value_to_string.vi"("precision"=w957, "Value"=w953, "Label for value"=w955) -> ("Output string"=w951:string)
            n389 = call "Value_to_string.vi"("precision"=w969, "Value"=w961, "Label for value"=w968) -> ("Output string"=w970:string)
            n390 = call "Value_to_string.vi"("precision"=w969, "Value"=w960, "Label for value"=w967) -> ("Output string"=w971:string)
            n391 = call "Value_to_string.vi"("precision"=w969, "Value"=w959, "Label for value"=w966) -> ("Output string"=w972:string)
            n392 = call "Value_to_string.vi"("precision"=w969, "Value"=w958, "Label for value"=w965) -> ("Output string"=w973:string)
            n393 = Concatenate Strings(w952, w951, w962, w970, w971, w972, w973, w962) -> (w963:string)
            n394 = global write "LDA_meas_global_1.vi" "Min Green Unshifted Power mW"(w961) -> ()
            n395 = global write "LDA_meas_global_1.vi" "Min Blue Unshifted Power mW"(w959) -> ()
            n396 = global write "LDA_meas_global_1.vi" "Min Green Shifted Power mW"(w960) -> ()
            n397 = global write "LDA_meas_global_1.vi" "Min Blue Shifted Power mW"(w958) -> ()
          }
          frame #2 {
            n398 = case shown="True" w974 {
              tunnel: w976 -> [_ w980]
              tunnel: w975 -> [_ w979]
              frame False {
              }
              frame True {
                n399 = local read "LDA_Probe_Information File"() -> (w983:path)
                n400 = local read "Channel Names"() -> (w982:string[])
                n401 = local read "Channel Values"() -> (w981:string[][])
                n402 = Current VI's Path() -> (path=w977:path)
                n403 = Initialize Array("", 15) -> (w986:string[])
                n404 = call "Open_Close_Front_Panel.ph.vi"("Front Panel Window:Open"=FALSE, "VI path"=w977) -> ()  [unwired: 2 out]
                n405 = call "Asterisk_header.vi"("Channel names"=w986) -> ("Header string"=w985:string)
                n406 = Concatenate Strings(w980, w979, w985) -> (w984:string)
                n407 = call "Write_Ch_data_file.vi"("Header string"=w984, "exists?"=FALSE, "Channel Values"=w981, "Channel names"=w982, "Filename"=w983) -> ()  [unwired: 2 in, 5 out]
              }
            }
          }
          frame #3 {
            n408 = local read "Probe Options"() -> (w990:string[])
            n409 = local read "Setup Array"() -> (w991:T3)
            n410 = for {
              tunnel: w991 -> [w1001] mode=indexing
              tunnel: w990 -> [w1000]
              i -> [w998]
              n411 = Unbundle By Name(w1001) -> ("Probe Type"=w999:u16)
              n412 = Index Array(array=w1000, index=w999) -> (element=w997:string)
              n413 = case shown="1" w998 {
                tunnel: w997 -> [w1002 w1003]
                frame 0, Default {
                  n414 = global write "LDA_meas_global_1.vi" "Probe Type"(w1002) -> ()
                }
                frame 1 {
                  n415 = global write "LDA_meas_global_2.vi" "Probe Type 2"(w1003) -> ()
                }
              }
            }
          }
        }
      }
    }
    n416 = case shown="No Error" w31 {
      tunnel: [w43 "Error"] -> w40
      tunnel: w39 -> [w43 _]
      frame No Error {
      }
      frame Error {
      }
    }
  }
